vi "Autonomous Independent.vi"() -> ()   [LabVIEW 2017]
doc: "This VI is called when autonomous begins, and will automatically be terminated when autonomous ends. You can carry out timed or sensor driven robot movement independently without needing to return to the caller."
uses:
  <vilib>/Rock Robotics/WPI/Utilities/WPI_GetSetVariantRefNum.vi
  <vilib>/Rock Robotics/Network Tables/NT Read String.vi
  <vilib>/Rock Robotics/Network Tables/NT Write Numeric Array.vi
  <vilib>/Rock Robotics/Network Tables/NT Write String.vi
  <vilib>/Rock Robotics/Network Tables/NT Write Number.vi
  <vilib>/Rock Robotics/Network Tables/NT Read Number.vi
  <vilib>/Rock Robotics/WPI/Ultrasonic/WPI_SonarMB1010AnalogRefNum Registry Get.vi
  <vilib>/addons/control/pid/NI_PID_pid.lvlib
  <vilib>/addons/control/pid/pid.llb/PID (DBL).vi
  <vilib>/Rock Robotics/WPI/Ultrasonic/WPI_SonarMB1010AnalogGetRange.vi
panel:
  out "Current Movement, for debugging":T1 {"Y Joystick Value" scale=1.0..-1.0; "X Joystick Value" scale=-1.0..1.0}
  in  "Array of robot movements":T2(array[cluster])=[{"X Joystick Value"=0.39393939393939403, "Y Joystick Value"=0.0, "Delay (sec)"=1.0, "Movement Name"="turn"}, {"X Joystick Value"=-0.3737373737373737, "Y Joystick Value"=0.0, "Delay (sec)"=1.0, "Movement Name"="turn back"}] {"Y Joystick Value" scale=1.0..-1.0; "X Joystick Value" scale=-1.0..1.0}
  # "Be sure to right-click and choose Data Operations>>Make Current Value default if you want to save the array values with the VI"
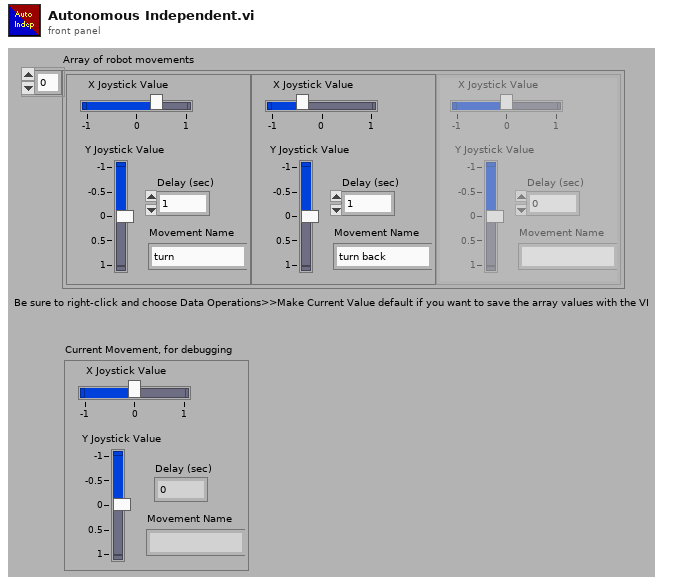
[diagram p1: front panel]
types:
  T1 = cluster{"X Joystick Value":dbl, "Y Joystick Value":dbl, "Delay (sec)":dbl, "Movement Name":string}
  T2 = cluster{"X Joystick Value":dbl, "Y Joystick Value":dbl, "Delay (sec)":dbl, "Movement Name":string}[]
  T3 = typedef "NetComm_MatchType.ctl" = enum32{"None", "Practice", "Qualification", "Elimination"}
  T4 = typedef "WPI_DriverStationPositionInfo.ctl" = enum16{"1", "2", "3"}
  T5 = typedef "WPI_DriverStationAllianceInfo.ctl" = enum16{"Red", "Blue", "Invalid"}
  T6 = typedef "WPI_JoystickDevRef.ctl" = cluster{"Device":T7}
  T7 = typedef "WPI_JoystickDeviceEnum.ctl" = enum16{"USB 0", "USB 1", "USB 2", "USB 3", "USB 4", "USB 5"}
  T8 = typedef "WPI_GyroDevRef.ctl" = cluster{"DevStatus":errorcluster, "Analog Channel":T9, "Gain (VoltsPerDegree/Second)":dbl, "Gyro Type":enum16{"Analog", "XRS450"}, "Handle":i32, "SPI Bus":T10, "Device Found":bool, "Sample Rate":dbl, "Calibrate On Open":bool, "Offset":dbl}
  T9 = typedef "FPGA_AIChannel.ctl" = enum8{"AI 0", "AI 1", "AI 2", "AI 3", "AI MXP 0", "AI MXP 1", "AI MXP 2", "AI MXP 3", "Invalid"}
  T10 = typedef "spi_bus.ctl" = enum16{"SPI On-Board, CS0", "SPI On-Board, CS1", "SPI On-Board, CS2", "SPI On-Board, CS3", "SPI MXP", "Invalid"}
  T11 = typedef "WPI_RobotDriveDevRef.ctl" = cluster{"DevStatus":errorcluster, "Motors[]":T12[], "Square Inputs":bool, "Max Output":dbl}
  T12 = typedef "WPI_MotorControlDeviceRef.ctl" = cluster{"DeviceStatus":errorcluster, "Type":T13, "PWM":cluster{"PWM Channel":T14, "DeadBand":T15}, "CAN":cluster{"Device Number":u8, "SetOutput VI Ref":variant, "GetOutput VI Ref":variant, "Enable VI Ref":variant, "Disable VI Ref":variant, "Data":variant}, "Invert":bool, "DIO PWM":cluster{"PWM \"Enable\" Channel":T14, "DIOChannel":T16, "PWM Rate":dbl}}
  T13 = typedef "WPI_MotorControlType.ctl" = enum16{"PWM", "CAN", "DIO PWM"}
  T14 = typedef "FPGA_DIOPWMChannel.ctl" = enum8{"PWM 0", "PWM 1", "PWM 2", "PWM 3", "PWM 4", "PWM 5", "PWM 6", "PWM 7", "PWM 8", "PWM 9", "PWM MXP 0", "PWM MXP 1", "PWM MXP 2", "PWM MXP 3", "PWM MXP 4", "PWM MXP 5", "PWM MXP 6", "PWM MXP 7", "PWM MXP 8", "PWM MXP 9", "Invalid"}
  T15 = typedef "WPI_PWMDeadband.ctl" = cluster{"Name":string, "maxPositivePwm":i32, "minPositivePwm":i32, "centerPwm":i32, "maxNegativePwm":i32, "minNegativePwm":i32, "angularRange":u16}
  T16 = typedef "FPGA_DIOChannel.ctl" = enum8{"DIO 0", "DIO 1", "DIO 2", "DIO 3", "DIO 4", "DIO 5", "DIO 6", "DIO 7", "DIO 8", "DIO 9", "DIO MXP 0", "DIO MXP 1", "DIO MXP 2", "DIO MXP 3", "DIO MXP 4", "DIO MXP 5", "DIO MXP 6", "DIO MXP 7", "DIO MXP 8", "DIO MXP 9", "DIO MXP 10", "DIO MXP 11", "DIO MXP 12", "DIO MXP 13", "DIO MXP 14", "DIO MXP 15", "SPI Port CS1", "SPI Port CS2", "SPI Port CS3", "SPI Port MISO", "SPI Port MOSI", "Invalid"}
  T17 = typedef "WPI_SonarMB1010AnalogDeviceRef.ctl" = cluster{"AIDeviceRef":T18, "Scaling factor (V/in)":dbl, "Average Bits":u8}
  T18 = typedef "WPI_AnalogChannelDevRef.ctl" = cluster{"DevStatus":errorcluster, "Analog Channel":T9}
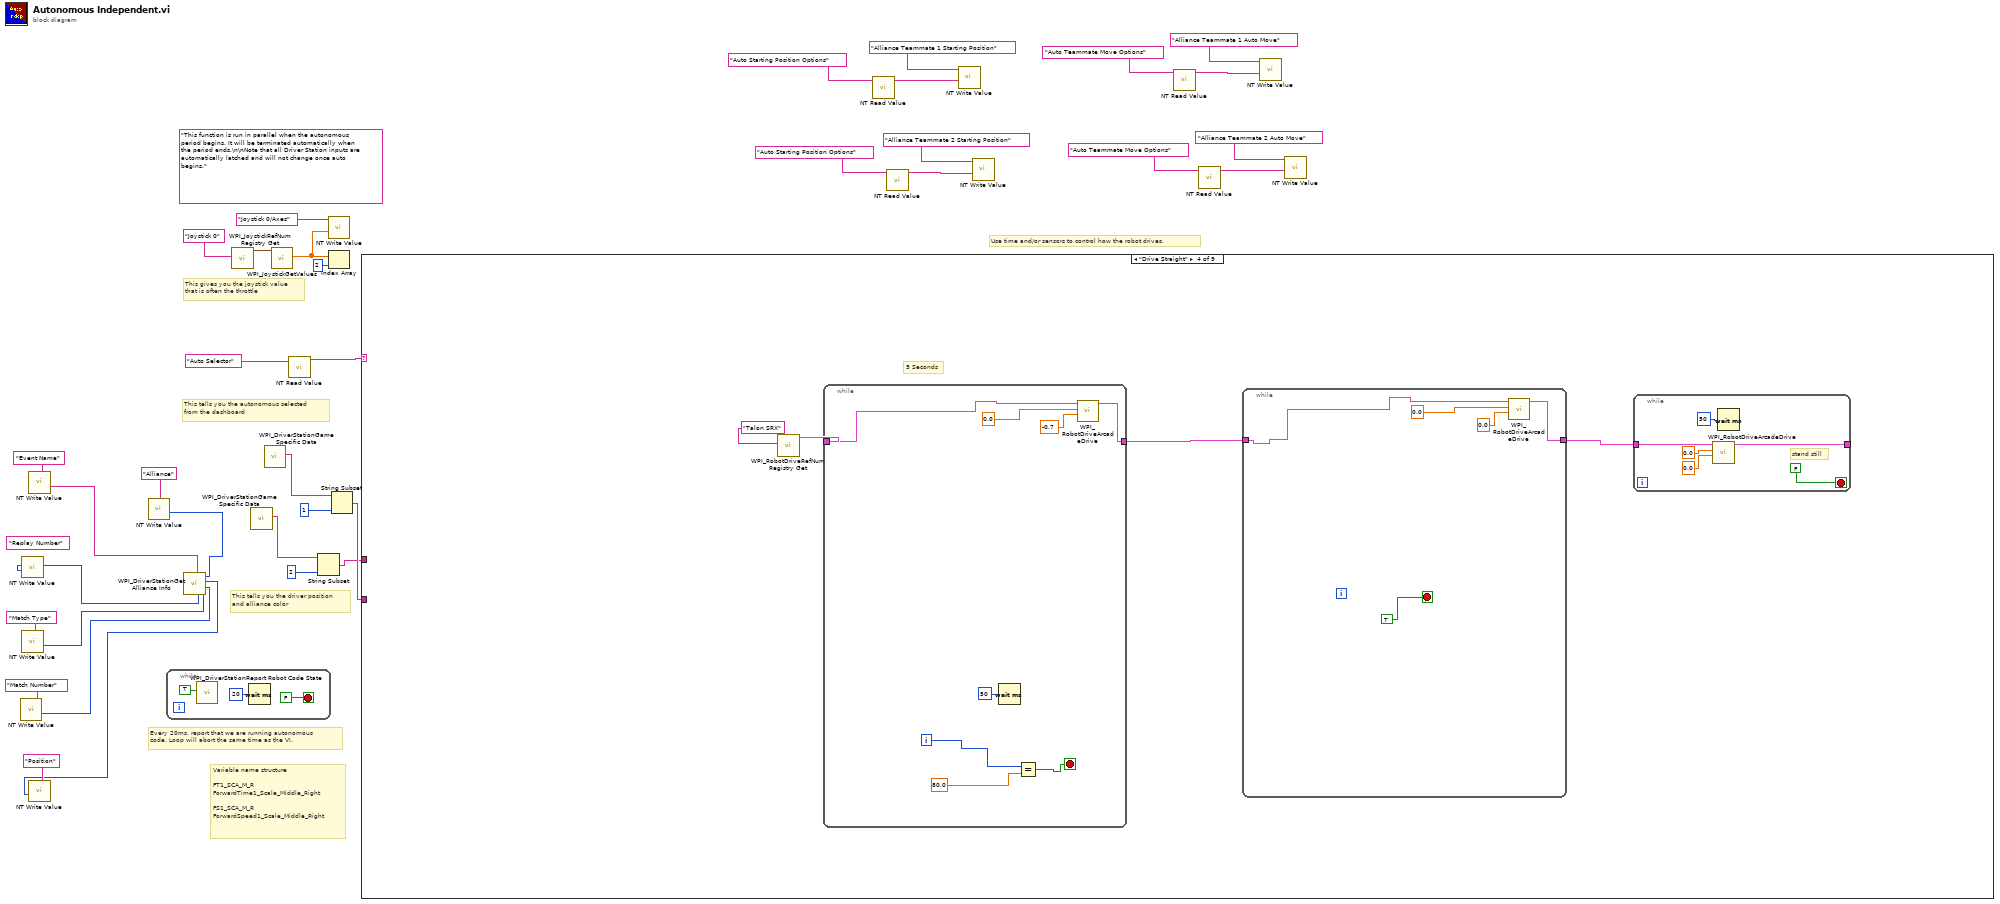
[diagram p0: block diagram]
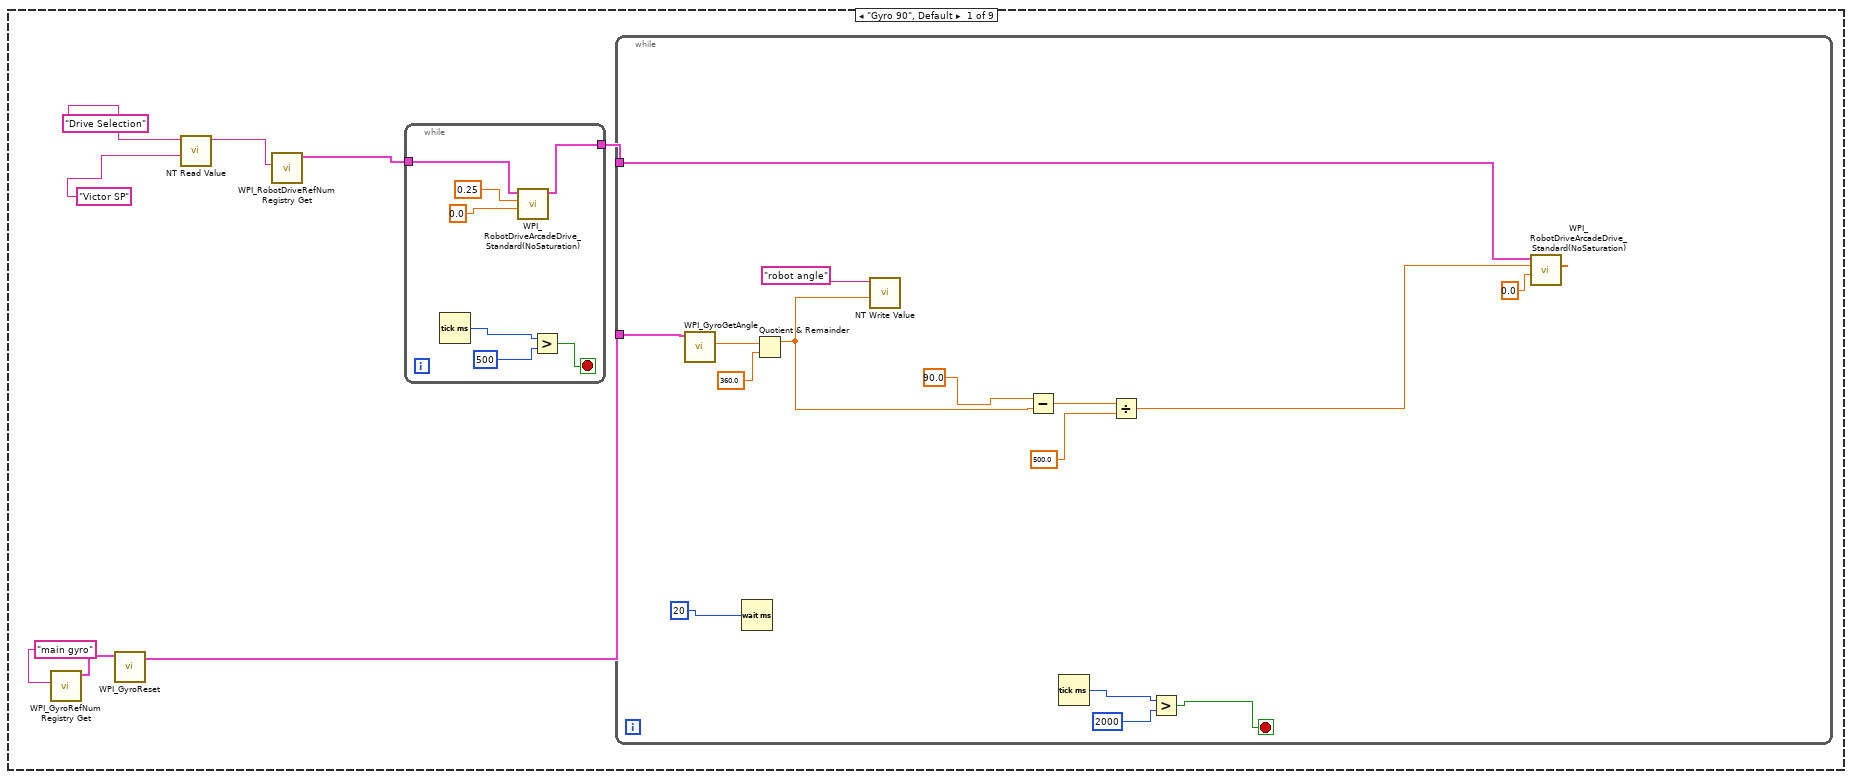
[diagram p2: hidden frame]
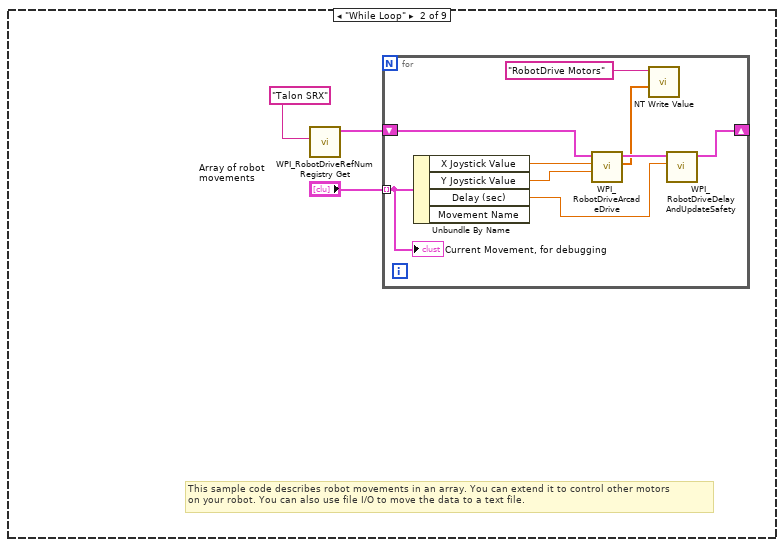
[diagram p3: hidden frame]
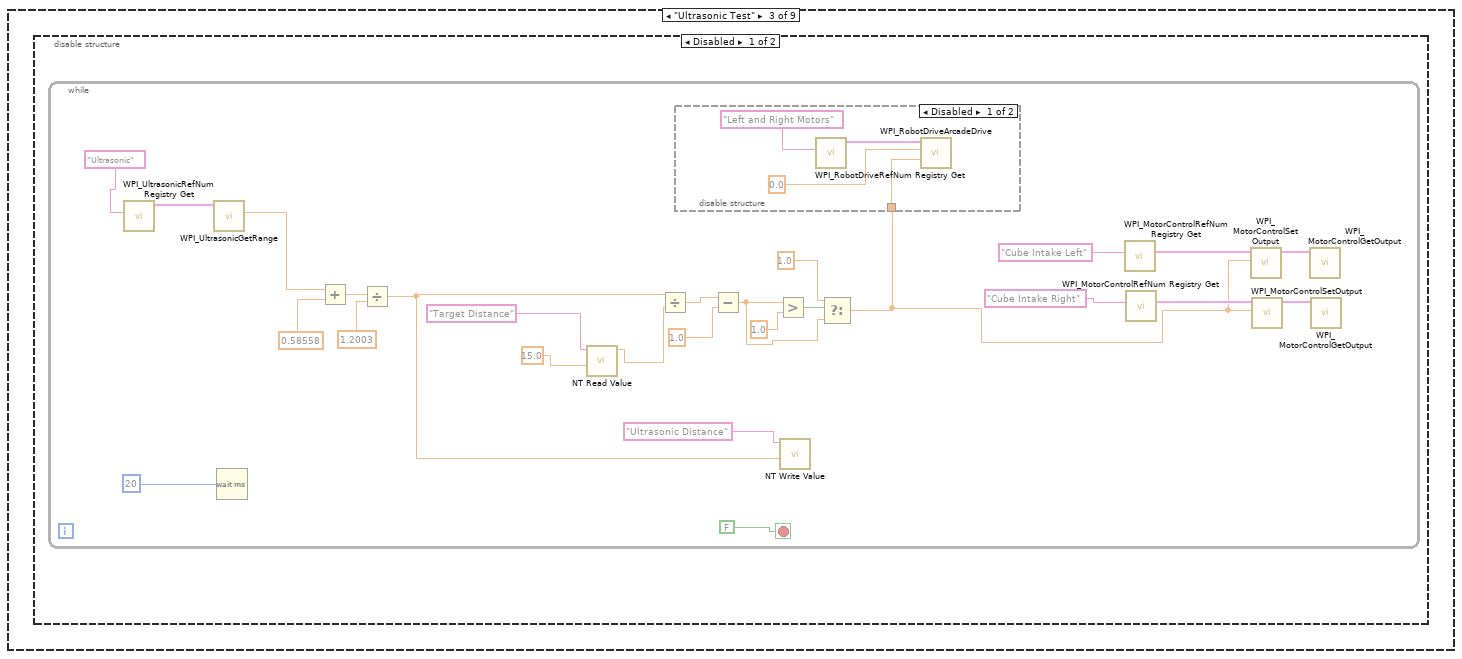
[diagram p4: hidden frame]
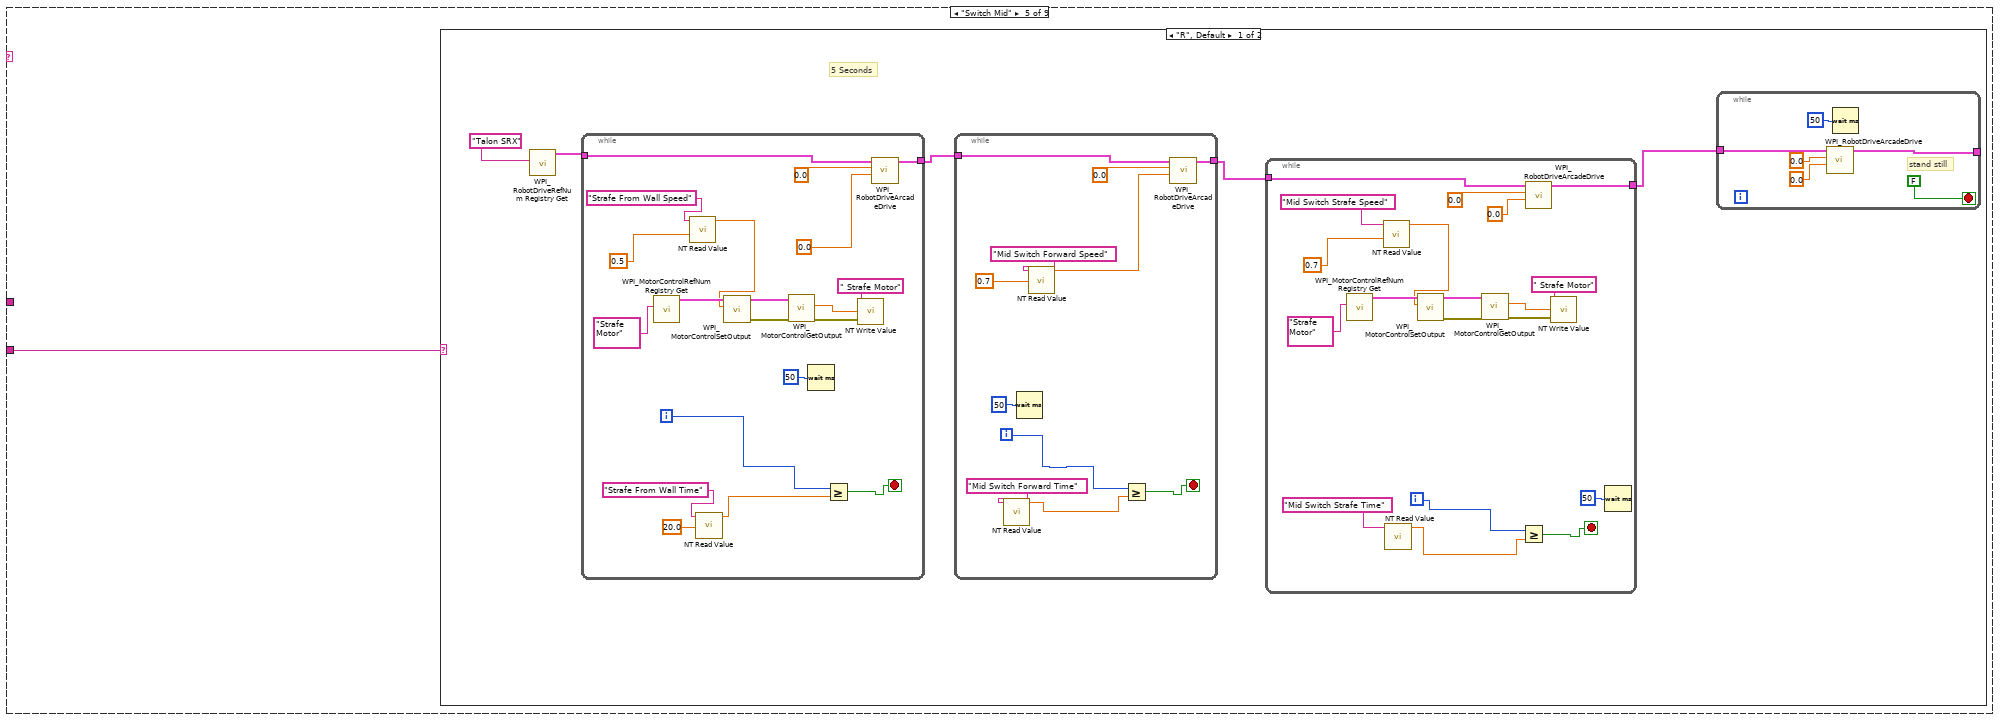
[diagram p7: hidden frame]
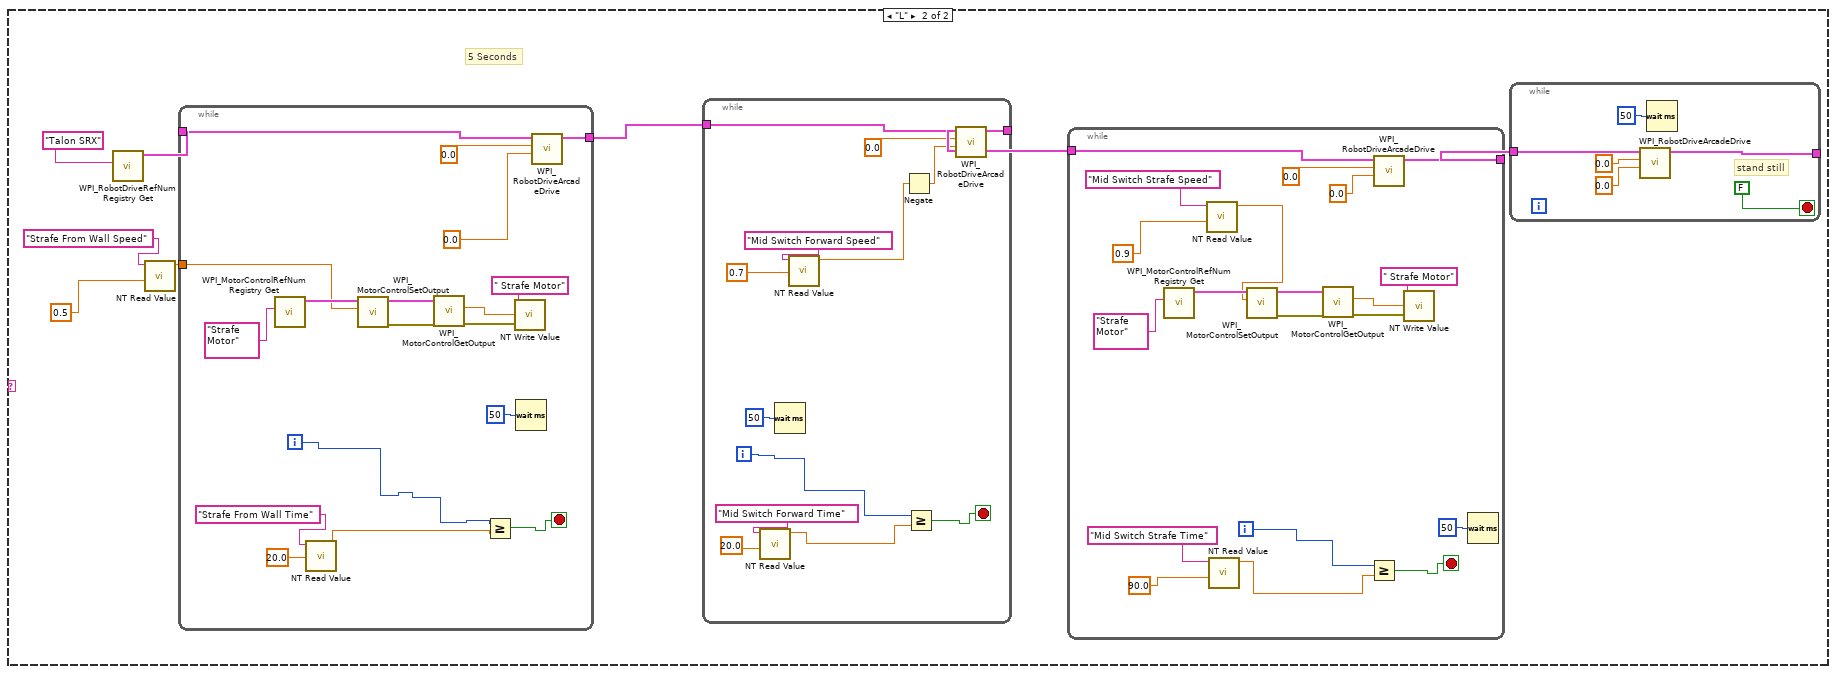
[diagram p8: hidden frame]
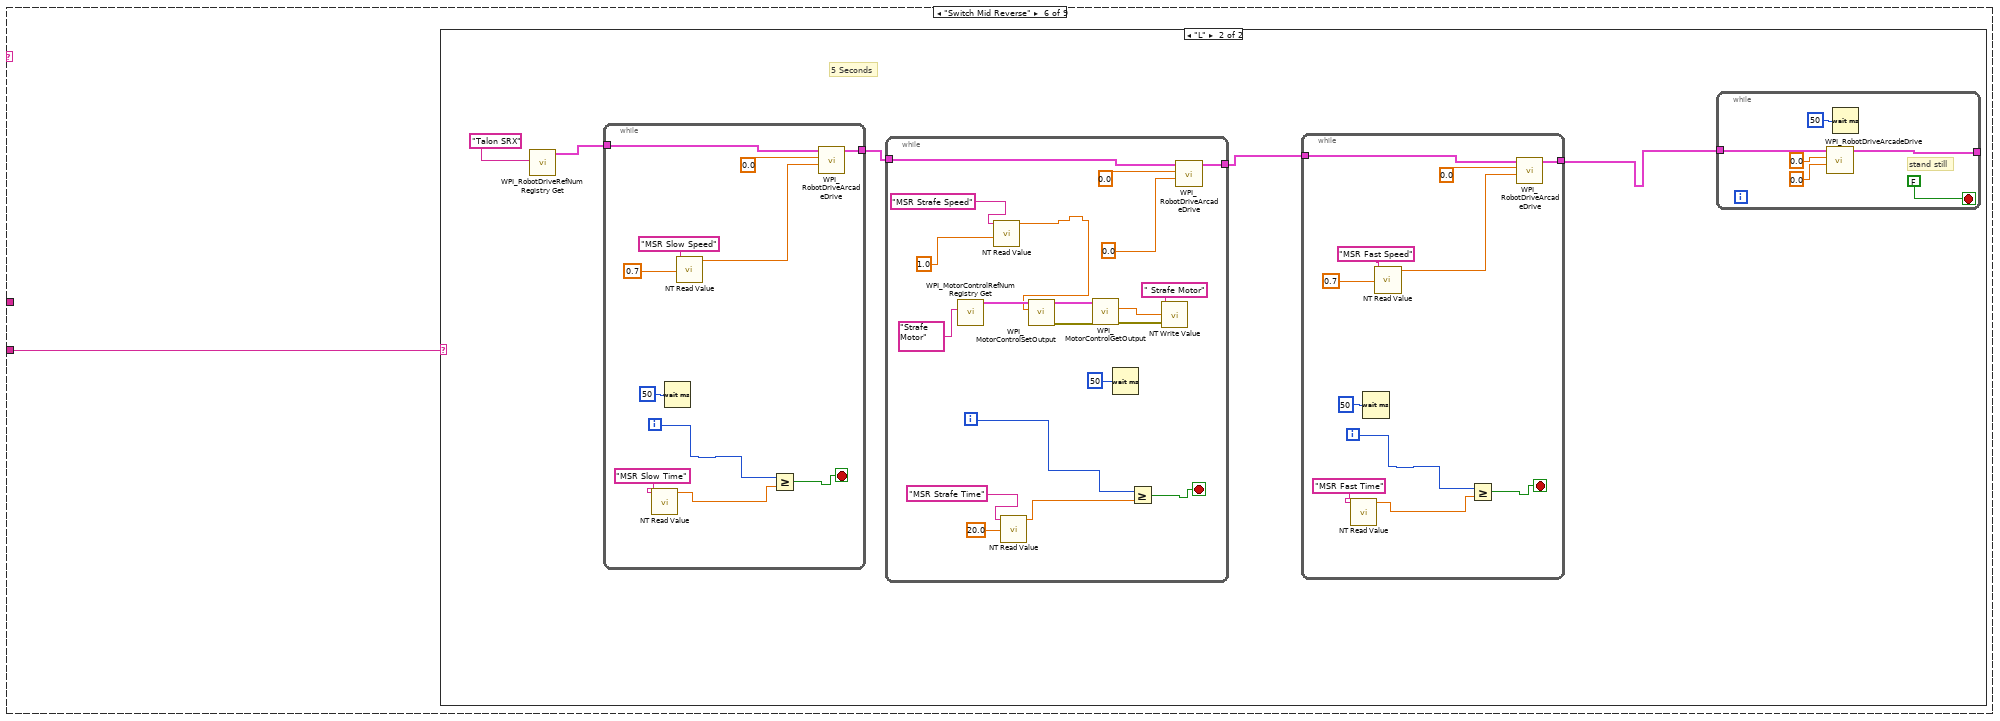
[diagram p9: hidden frame]
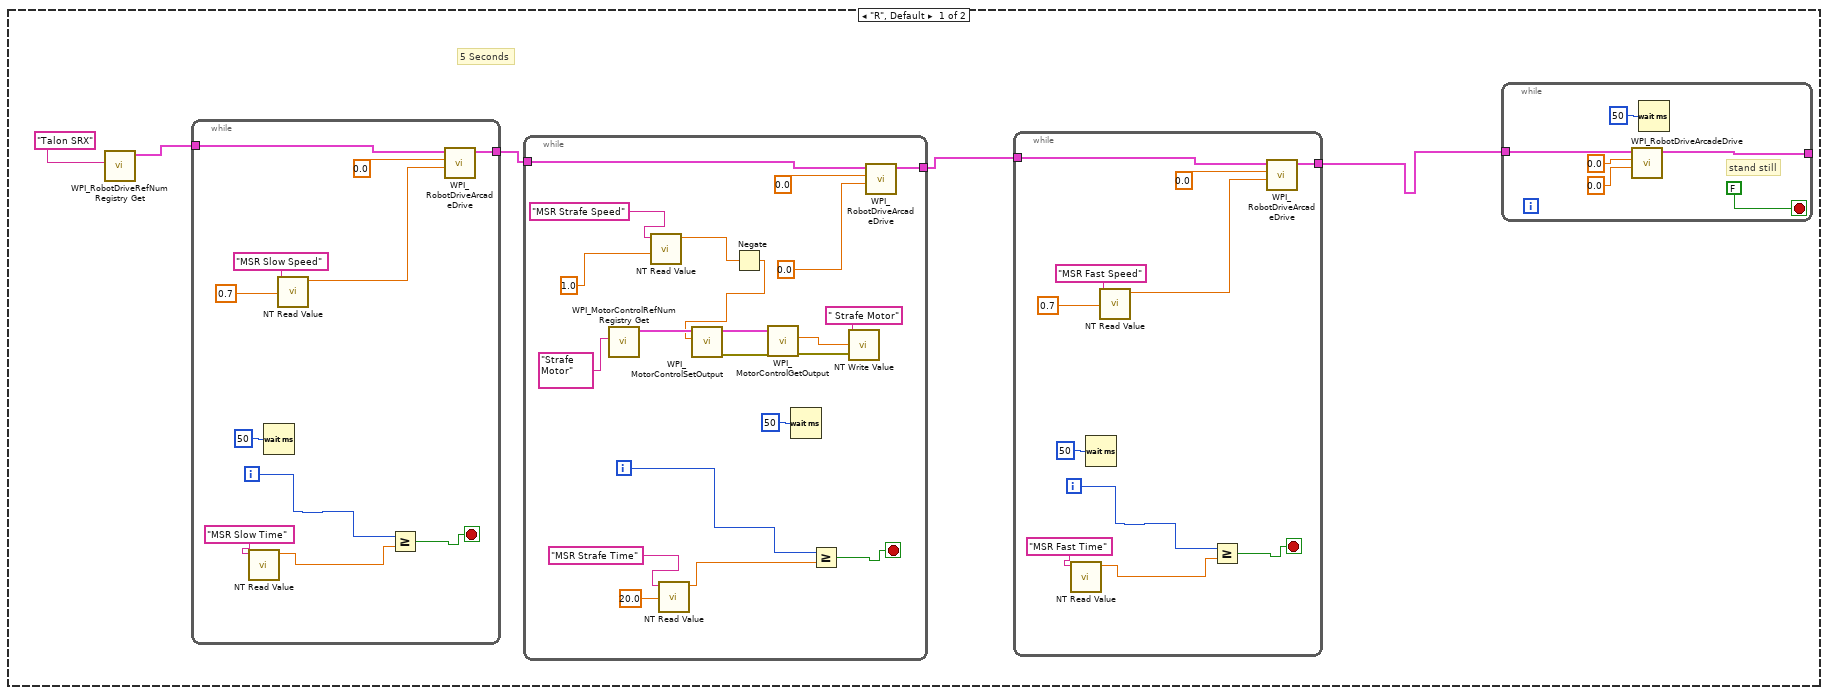
[diagram p10: hidden frame]
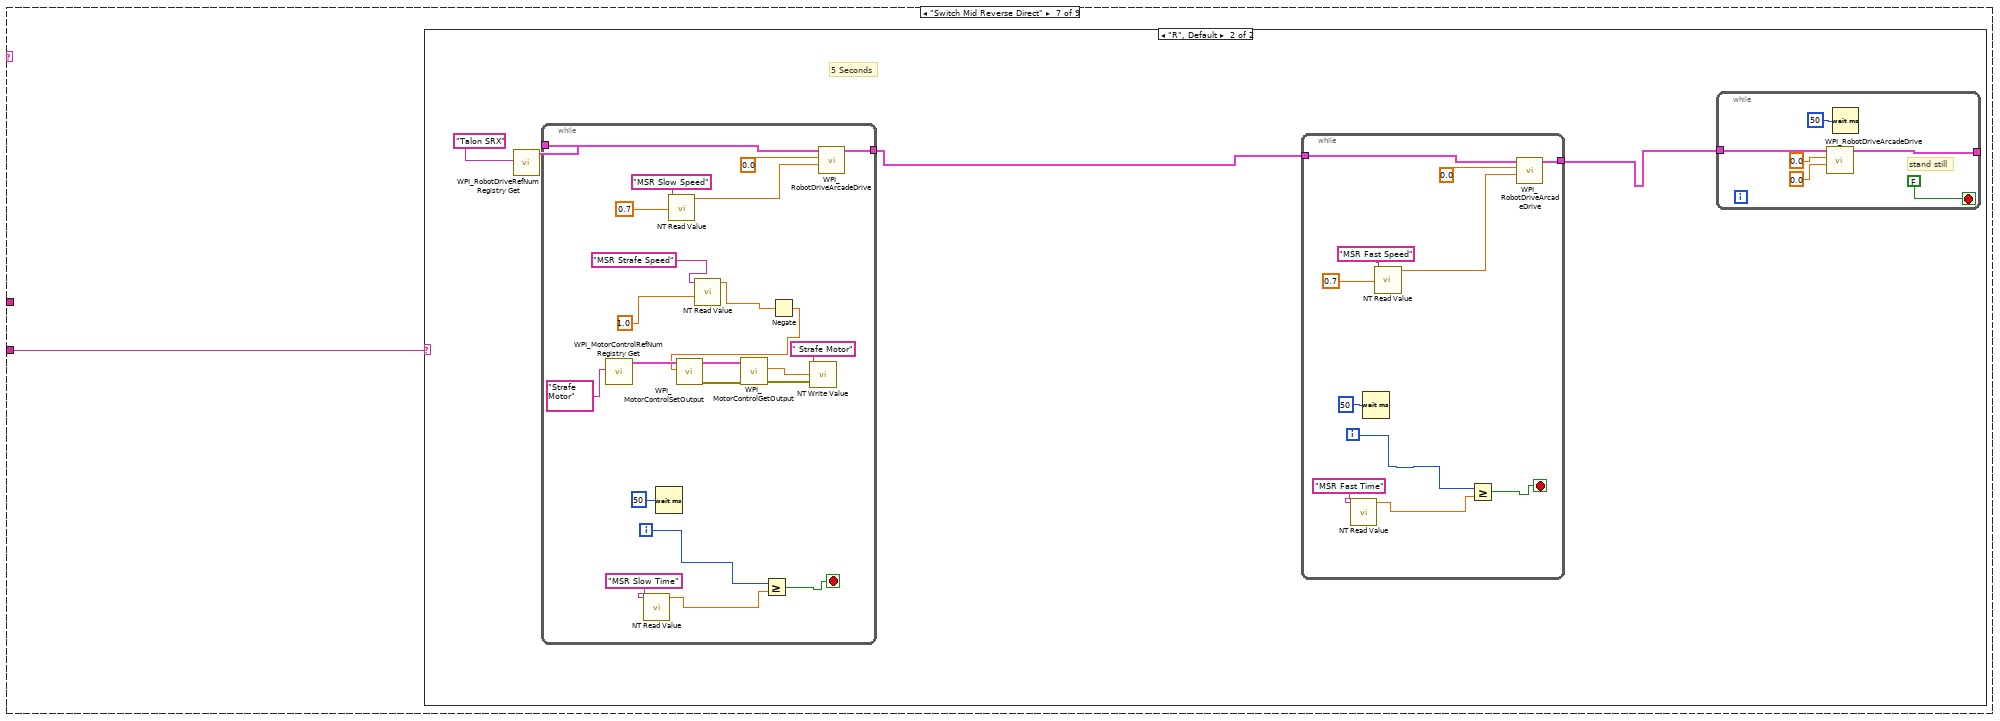
[diagram p11: hidden frame]
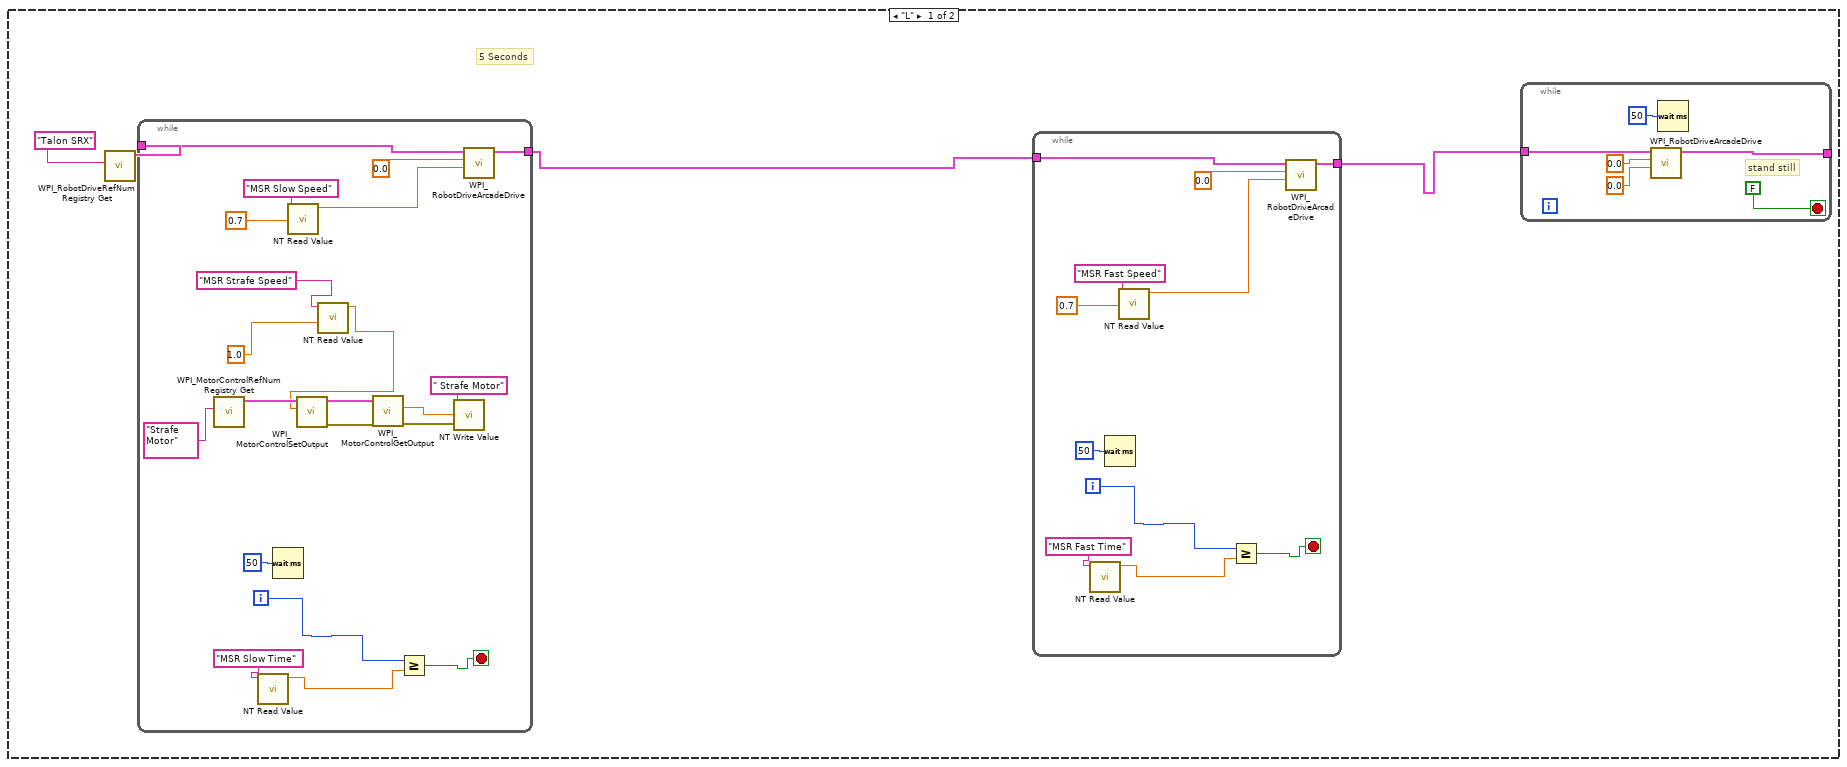
[diagram p12: hidden frame]
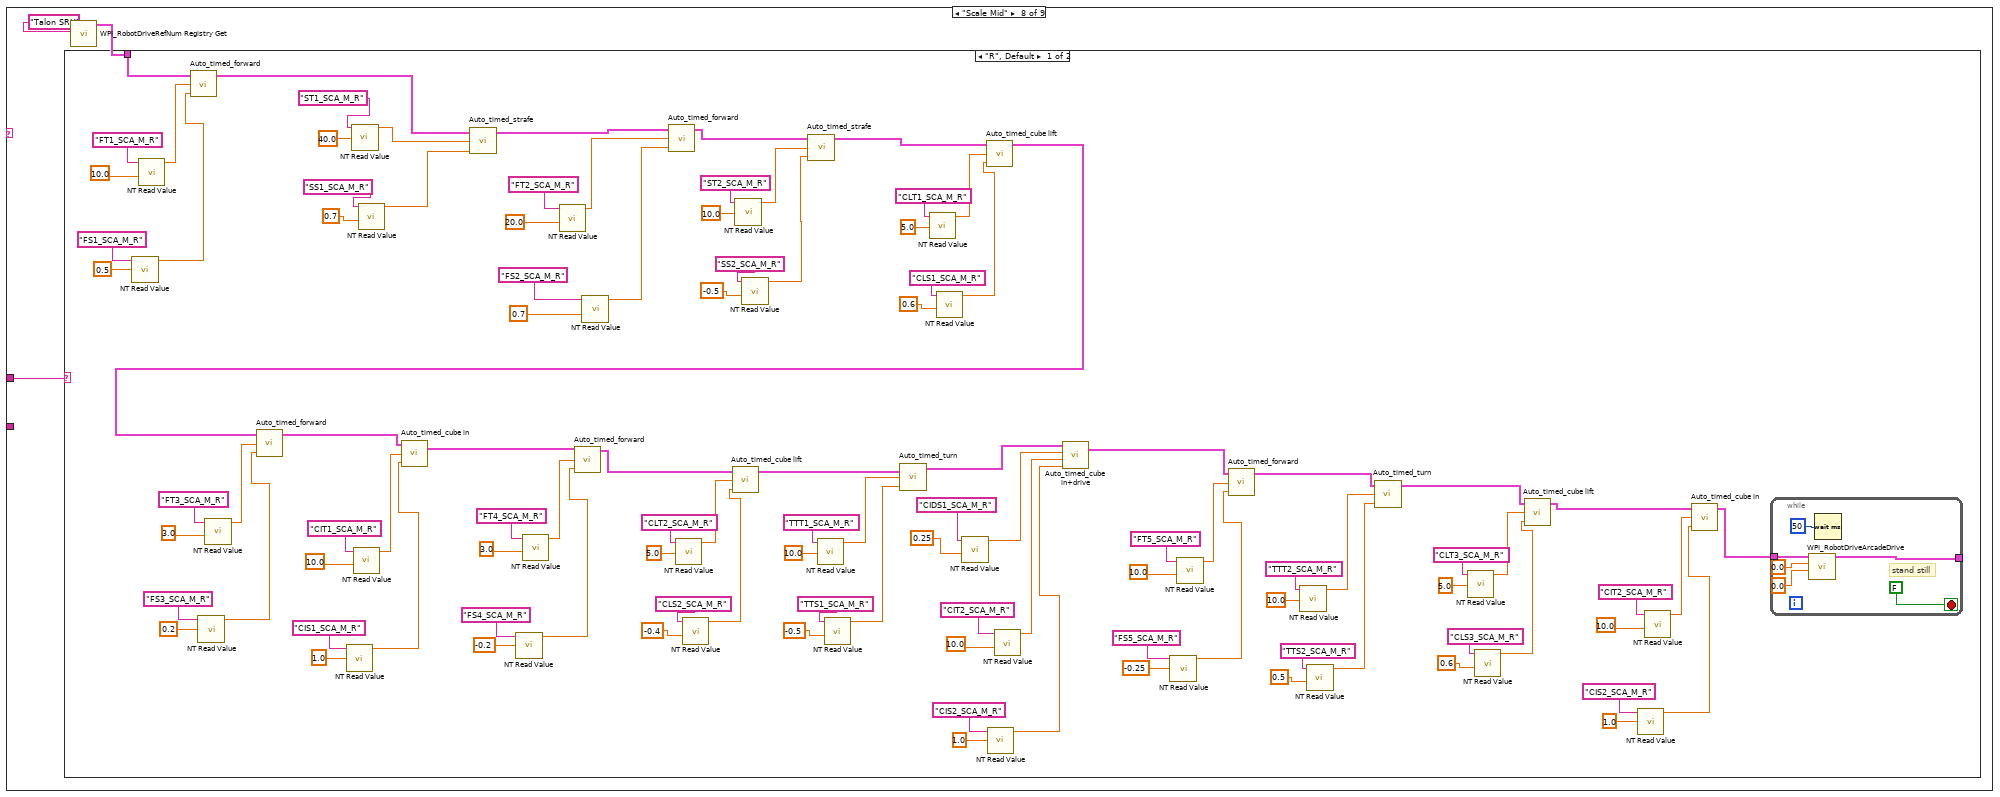
[diagram p13: hidden frame]
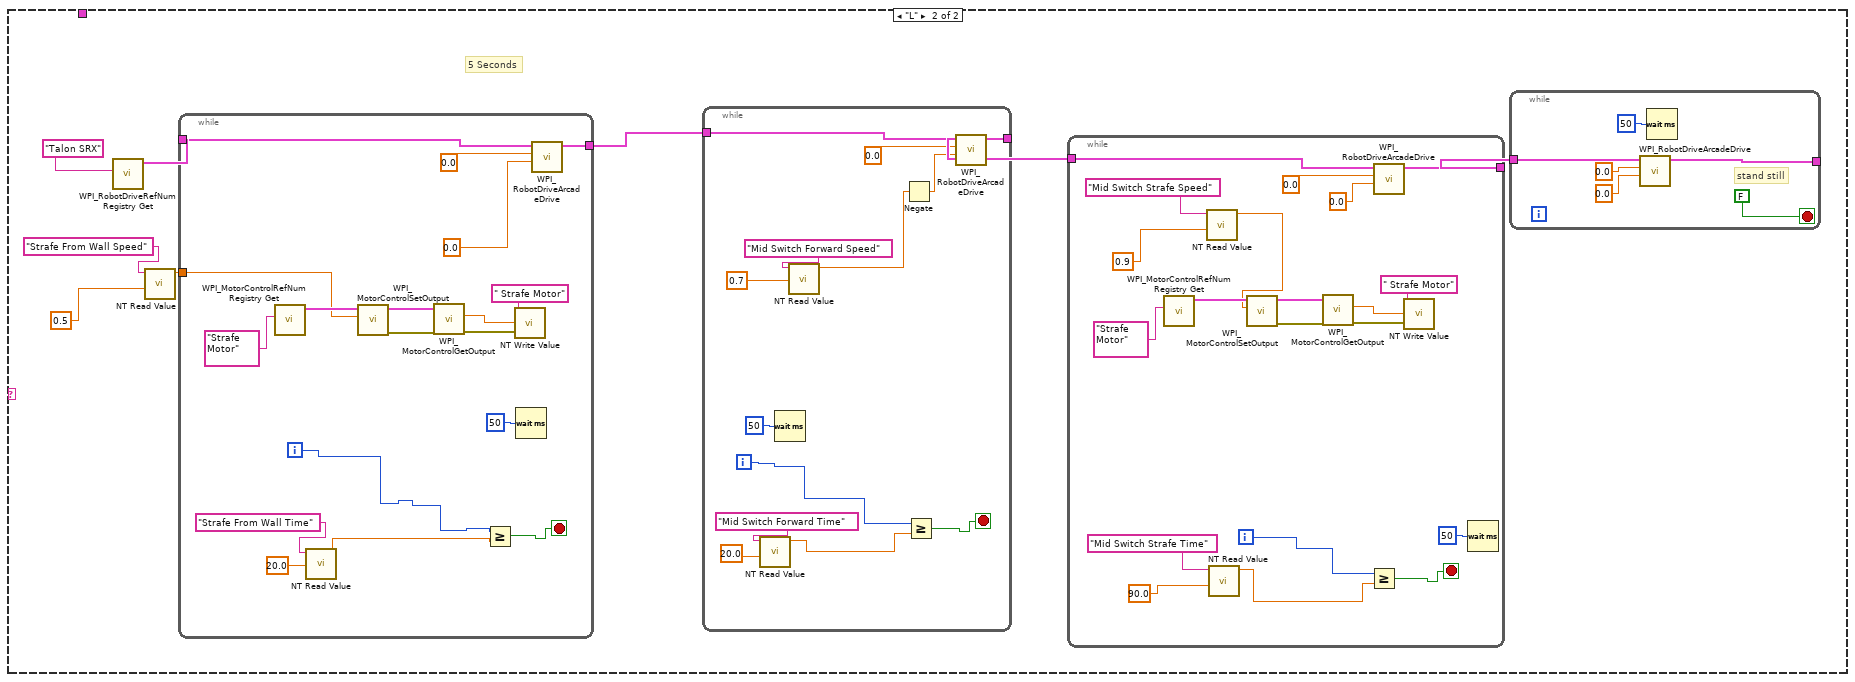
[diagram p14: hidden frame]
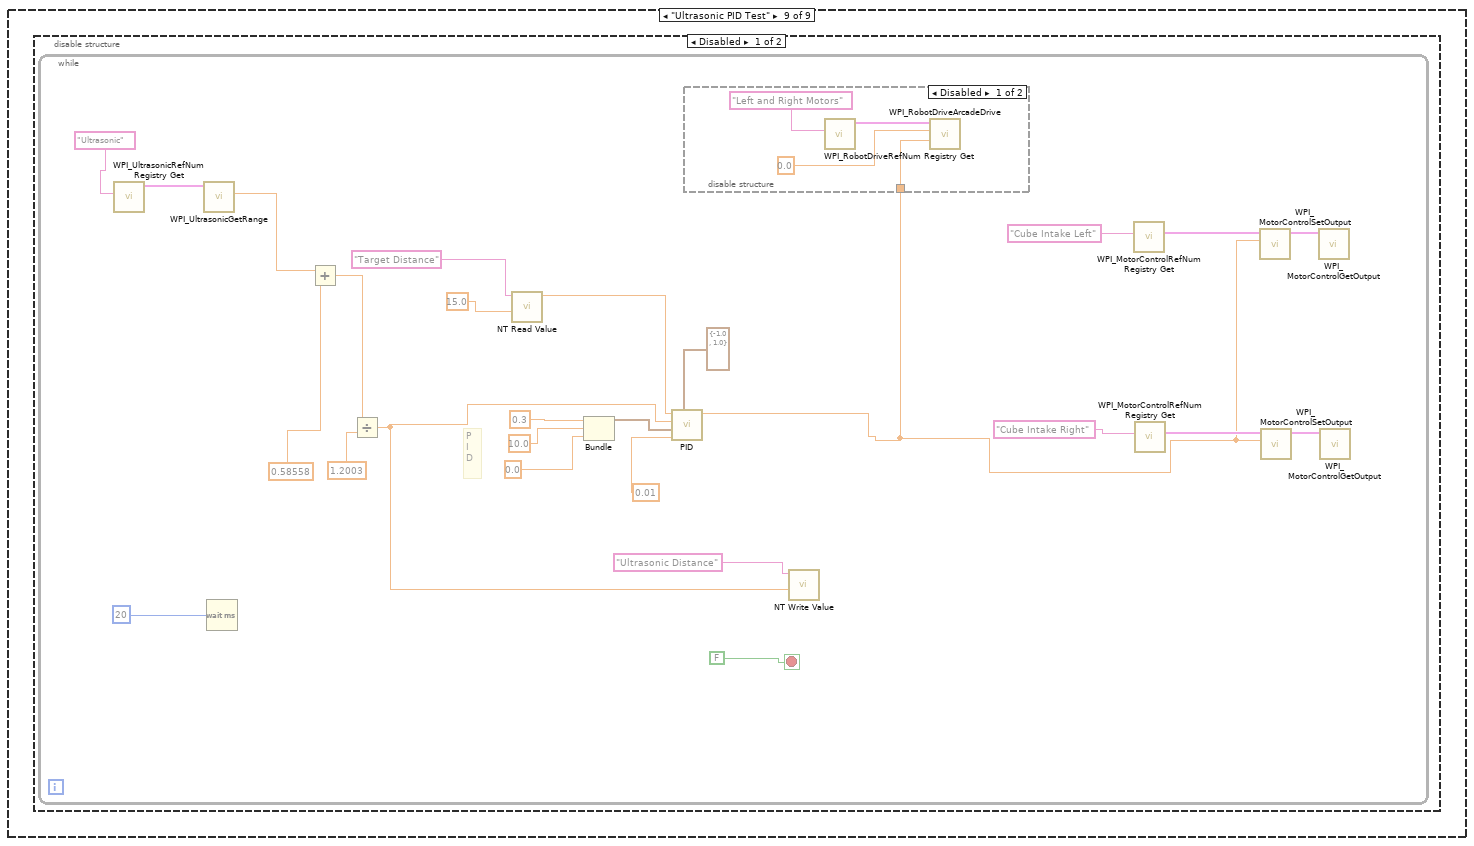
[diagram p15: hidden frame]
diagram:
  (unwired) "Replay Number"
  (unwired) "This function is run in parallel when the autonomous period begins. It will be terminated automatically when the period ends.\n\nNote that all Driver Station inputs are automatically latched and will not change once auto begins."
  # "Variable name structure\n\nFT1_SCA_M_R\nForwardTime1_Scale_Middle_Right\n\nFS1_SCA_M_R\nForwardSpeed1_Scale_Middle_Right"
  # "This tells you the autonomous selected\nfrom the dashboard"
  # "Every 20ms, report that we are running autonomous\ncode. Loop will abort the same time as the VI."
  # "This gives you the joystick value\nthat is often the throttle"
  # "Use time and/or sensors to control how the robot drives."
  # "This tells you the driver position\nand alliance color"
  n1 = while {
    stop <- FALSE stop-if-true
    n2 = call <vilib>:"WPI_DriverStationReport Robot Code State.vi"("Autonomous"=TRUE) -> ()  [unwired: 10 in, 1 out]
    n3 = Wait (ms)(milliseconds to wait=u32 20) -> ()  [unwired: 1 out]
  }
  n4 = call <vilib>:"WPI_DriverStationGet Alliance Info.vi"() -> ("Match Type"=w17:T3, "Match Number"=w18:u16, "Position"=w19:T4, "Alliance"=w23:T5, "Replay Number"=w16:u16, "Event Name"=w25:string)  [unwired: 6 out]
  n5 = call-poly <vilib>:"NT Write Value.vi"("Numeric"=w18, "Name"="Match Number") -> ()  [unwired: 9 in, 1 out]
  n6 = call-poly <vilib>:"NT Write Value.vi"("Numeric"=w16) -> ()  [unwired: 10 in, 1 out]
  n7 = call-poly <vilib>:"NT Write Value.vi"("Numeric"=w17, "Name"="Match Type") -> ()  [unwired: 9 in, 1 out]
  n8 = call-poly <vilib>:"NT Write Value.vi"("String"=w25, "Name"="Event Name") -> ()  [unwired: 9 in, 1 out]
  n9 = call-poly <vilib>:"NT Write Value.vi"("Numeric"=w19, "Name"="Position") -> ()  [unwired: 9 in, 1 out]
  n10 = call-poly <vilib>:"NT Write Value.vi"("Numeric"=w23, "Name"="Alliance") -> ()  [unwired: 9 in, 1 out]
  n11 = call <vilib>:"WPI_JoystickRefNum Registry Get.vi"("refnum name"="Joystick 0") -> ("JoystickDevRef"=w35:T6)  [unwired: 1 in, 9 out]
  n12 = call <vilib>:"WPI_DriverStationGame Specific Data.vi"() -> ("Game Specific Data"=w3:string)  [unwired: 11 in]
  n13 = call <vilib>:"WPI_DriverStationGame Specific Data.vi"() -> ("Game Specific Data"=w29:string)  [unwired: 11 in]
  n14 = call <vilib>:"WPI_JoystickGetValues.vi"("JoystickDevRef"=w35) -> ("Axes"=w31:dbl[])  [unwired: 6 in, 4 out]
  n15 = call-poly <vilib>:"NT Read Value.vi"("Name"="Auto Selector") -> ("String"=w32:string)  [unwired: 9 in, 1 out]
  n16 = String Subset(string=w3, length (rest)=2 ("index")) -> (substring=w1:string)  [unwired: 1 in]
  n17 = call-poly <vilib>:"NT Write Value.vi"("Numeric Array"=w31, "Name"="Joystick 0/Axes") -> ()  [unwired: 9 in, 1 out]
  n18 = Index Array(array=w31, index=2) -> ()  [unwired: 1 out]
  n19 = String Subset(string=w29, length (rest)=1 ("index")) -> (substring=w28:string)  [unwired: 1 in]
  n20 = case shown="\"Drive Straight\"" w32 {
    tunnel: w28 -> [_ _ _ _ w135 w262 w370 _ _]
    tunnel: w1 -> [_ _ _ _ _ _ _ w456 _]
    frame "Gyro 90", Default {
      n21 = call <vilib>:"WPI_GyroRefNum Registry Get.vi"("refnum name"="main gyro") -> ("GyroDevRef"=w45:T8)  [unwired: 9 in, 1 out]
      n22 = call <vilib>:"WPI_GyroReset.vi"("GyroDevRef"=w45) -> ("GyroDevRef"=w47:T8)  [unwired: 9 in, 1 out]
      n23 = call-poly <vilib>:"NT Read Value.vi"("Default Value"="Victor SP", "Name"="Drive Selection") -> ("String"=w44:string)  [unwired: 8 in, 1 out]
      n24 = call <vilib>:"WPI_RobotDriveRefNum Registry Get.vi"("refnum name"=w44) -> ("RobotDriveDevRef"=w41:T11)  [unwired: 1 in, 9 out]
      n25 = while {
        tunnel: w41 -> [w51]
        tunnel: [w48] -> w40
        stop <- w52 stop-if-true
        n26 = Tick Count (ms)() -> (millisecond timer value=w53:u32)
        n27 = call <vilib>:"WPI_RobotDriveArcadeDrive_Standard(NoSaturation).vi"("Y axis value"=0.0, "X axis value"=0.25, "RobotDriveDevRef"=w51) -> ("RobotDriveDevRef"=w48:T11)  [unwired: 1 in, 7 out]
        n28 = Greater?(x=w53, y=500) -> (0:w52:bool)
      }
      n29 = while {
        tunnel: w47 -> [w66]
        tunnel: w40 -> [w63]
        stop <- w62 stop-if-true
        n30 = call <vilib>:"WPI_GyroGetAngle.vi"("GyroDevRef"=w66) -> ("Angle"=w67:dbl)  [unwired: 6 in, 4 out]
        n31 = Wait (ms)(milliseconds to wait=u32 20) -> ()  [unwired: 1 out]
        n32 = Quotient & Remainder(x=w67, y=360.0) -> (x-y*floor(x/y)=w58:dbl)  [unwired: 1 out]
        n33 = call-poly <vilib>:"NT Write Value.vi"("Numeric"=w58, "Name"="robot angle") -> ()  [unwired: 9 in, 1 out]
        n34 = Subtract(x=90.0, y=w58) -> (x-y=w57:dbl)
        n35 = Tick Count (ms)() -> (millisecond timer value=w60:u32)
        n36 = Divide(x=w57, y=500.0) -> (x/y=w55:dbl)
        n37 = Greater?(x=w60, y=2000) -> (0:w62:bool)
        n38 = call <vilib>:"WPI_RobotDriveArcadeDrive_Standard(NoSaturation).vi"("Y axis value"=0.0, "X axis value"=w55, "RobotDriveDevRef"=w63) -> ()  [unwired: 1 in, 8 out]
      }
    }
    frame "While Loop" {
      # "This sample code describes robot movements in an array. You can extend it to control other motors\non your robot. You can also use file I/O to move the data to a text file."
      n39 = call <vilib>:"WPI_RobotDriveRefNum Registry Get.vi"("refnum name"="Talon SRX") -> ("RobotDriveDevRef"=w71:T11)  [unwired: 1 in, 9 out]
      n40 = for {
        shift-right: [w79] -> _
        shift-left: w71 -> [w80]
        tunnel: "Array of robot movements" -> [w75] mode=indexing
        n41 = Unbundle By Name(w75) -> ("X Joystick Value"=w78:dbl, "Y Joystick Value"=w77:dbl, "Delay (sec)"=w76:dbl)  [unwired: 1 out]
        n42 = call-poly <vilib>:"WPI_RobotDriveArcadeDrive.vi"("Y axis value"=w77, "X axis value"=w78, "RobotDriveDevRef"=w80) -> ("Motor Values"=w73:dbl[], "RobotDriveDevRef"=w81:T11)  [unwired: 1 in, 6 out]
        n43 = call-poly <vilib>:"NT Write Value.vi"("Numeric Array"=w73, "Name"="RobotDrive Motors") -> ()  [unwired: 9 in, 1 out]
        n44 = call <vilib>:"WPI_RobotDriveDelayAndUpdateSafety.vi"("Delay (s)"=w76, "RobotDriveDevRef"=w81) -> ("RobotDriveDevRef 2"=w79:T11)  [unwired: 8 in, 1 out]
        "Current Movement, for debugging" <- w75
      }
    }
    frame "Ultrasonic Test" {
      n45 = disable-structure shown="Disabled" {
        frame Disabled {
          n46 = while {
            stop <- FALSE stop-if-true
            n47 = call-poly <vilib>:"WPI_UltrasonicRefNum Registry Get.vi"("refnum name"="Ultrasonic") -> ("SonarMB1010AnalogDevRef"=w106:T17)  [unwired: 9 in, 1 out]
            n48 = call-poly <vilib>:"WPI_UltrasonicGetRange.vi"("SonarMB1010AnalogDevRef"=w106) -> ("Distance"=w105:dbl)  [unwired: 8 in, 2 out]
            n49 = Wait (ms)(milliseconds to wait=u32 20) -> ()  [unwired: 1 out]
            n50 = Add(x=w105, y=0.58558) -> (x+y=w103:dbl)
            n51 = Divide(x=w103, y=1.2003) -> (x/y=w95:dbl)
            n52 = call-poly <vilib>:"NT Read Value.vi"("Default Value"=15.0, "Name"="Target Distance" ("refnum name")) -> ("Numeric"=w85:dbl)  [unwired: 8 in, 1 out]
            n53 = Divide(x=w95, y=w85) -> (x/y=w100:dbl)
            n54 = Subtract(x=w100, y=1.0) -> (x-y=w96:dbl)
            n55 = Greater?(x=w96, y=1.0) -> (0:w99:bool)
            n56 = call-poly <vilib>:"NT Write Value.vi"("Numeric"=w95, "Name"="Ultrasonic Distance" ("refnum name")) -> ()  [unwired: 9 in, 1 out]
            n57 = Select(t=1.0, s=w99, f=w96) -> (s? t:f=w86:dbl)
            n58 = disable-structure shown="Disabled" {
              disable-tunnel: w86 -> [w108 _]
              frame Disabled {
                n59 = call <vilib>:"WPI_RobotDriveRefNum Registry Get.vi"("refnum name"="Left and Right Motors") -> ("RobotDriveDevRef"=w110:T11)  [unwired: 1 in, 9 out]
                n60 = call-poly <vilib>:"WPI_RobotDriveArcadeDrive.vi"("Y axis value"=w108, "X axis value"=0.0, "RobotDriveDevRef"=w110) -> ()  [unwired: 1 in, 8 out]
              }
              frame Enabled {
              }
            }
            n61 = call <vilib>:"WPI_MotorControlRefNum Registry Get.vi"("refnum name"="Cube Intake Left") -> ("MotorControlDevRef"=w89:T12)  [unwired: 9 in, 1 out]
            n62 = call <vilib>:"WPI_MotorControlRefNum Registry Get.vi"("refnum name"="Cube Intake Right") -> ("MotorControlDevRef"=w92:T12)  [unwired: 9 in, 1 out]
            n63 = call <vilib>:"WPI_MotorControlSetOutput.vi"("Output"=w86, "MotorControlDevRef"=w89) -> ("MotorControlDevRef"=w90:T12)  [unwired: 7 in, 2 out]
            n64 = call <vilib>:"WPI_MotorControlSetOutput.vi"("Output"=w86, "MotorControlDevRef"=w92) -> ("MotorControlDevRef"=w91:T12)  [unwired: 7 in, 2 out]
            n65 = call <vilib>:"WPI_MotorControlGetOutput.vi"("MotorControlDevRef"=w90) -> ()  [unwired: 8 in, 3 out]
            n66 = call <vilib>:"WPI_MotorControlGetOutput.vi"("MotorControlDevRef"=w91) -> ()  [unwired: 8 in, 3 out]
          }
        }
        frame Enabled {
        }
      }
    }
    frame "Drive Straight" {
      # "5 Seconds"
      n67 = call <vilib>:"WPI_RobotDriveRefNum Registry Get.vi"("refnum name"="Talon SRX") -> ("RobotDriveDevRef"=w114:T11)  [unwired: 1 in, 9 out]
      n68 = while {
        tunnel: w114 -> [w122]
        tunnel: [w121] -> w113
        i -> [w117]
        stop <- w116 stop-if-true
        n69 = Wait (ms)(milliseconds to wait=50) -> ()  [unwired: 1 out]
        n70 = Equal?(x=w117, y=80.0) -> (x = y?=w116:bool)
        n71 = call-poly <vilib>:"WPI_RobotDriveArcadeDrive.vi"("Y axis value"=-0.7 ("X axis value"), "X axis value"=0.0, "RobotDriveDevRef"=w122) -> ("RobotDriveDevRef"=w121:T11)  [unwired: 1 in, 7 out]
      }
      n72 = while {
        tunnel: w113 -> [w133]
        tunnel: [w132] -> w112
        stop <- TRUE stop-if-true
        n73 = call-poly <vilib>:"WPI_RobotDriveArcadeDrive.vi"("Y axis value"=0.0 ("X axis value"), "X axis value"=0.0, "RobotDriveDevRef"=w133) -> ("RobotDriveDevRef"=w132:T11)  [unwired: 1 in, 7 out]
      }
      n74 = while {
        tunnel: w112 -> [w125]
        tunnel: [w124] -> _
        stop <- FALSE stop-if-true
        # "stand still"
        n75 = call-poly <vilib>:"WPI_RobotDriveArcadeDrive.vi"("Y axis value"=0.0 ("X axis value"), "X axis value"=0.0, "RobotDriveDevRef"=w125) -> ("RobotDriveDevRef"=w124:T11)  [unwired: 1 in, 7 out]
        n76 = Wait (ms)(milliseconds to wait=50) -> ()  [unwired: 1 out]
      }
    }
    frame "Switch Mid" {
      n77 = case shown="\"R\", Default" w135 {
        frame "R", Default {
          # "5 Seconds"
          n78 = call <vilib>:"WPI_RobotDriveRefNum Registry Get.vi"("refnum name"="Talon SRX") -> ("RobotDriveDevRef"=w137:T11)  [unwired: 1 in, 9 out]
          n79 = while {
            tunnel: [w160] -> w136
            tunnel: w137 -> [w156]
            i -> [w147]
            stop <- w159 stop-if-true
            n80 = call <vilib>:"WPI_MotorControlRefNum Registry Get.vi"("refnum name"="Strafe Motor") -> ("MotorControlDevRef"=w153:T12)  [unwired: 9 in, 1 out]
            n81 = call-poly <vilib>:"NT Read Value.vi"("Default Value"=0.5 ("X axis value"), "Name"="Strafe From Wall Speed") -> ("Numeric"=w141:dbl)  [unwired: 8 in, 1 out]
            n82 = call-poly <vilib>:"NT Read Value.vi"("Default Value"=20.0 ("X axis value"), "Name"="Strafe From Wall Time") -> ("Numeric"=w144:dbl)  [unwired: 8 in, 1 out]
            n83 = call <vilib>:"WPI_MotorControlSetOutput.vi"("Output"=w141, "MotorControlDevRef"=w153) -> ("error out"=w151:errorcluster, "MotorControlDevRef"=w152:T12)  [unwired: 7 in, 1 out]
            n84 = call <vilib>:"WPI_MotorControlGetOutput.vi"("error in"=w151, "MotorControlDevRef"=w152) -> ("error out"=w149:errorcluster, "Output"=w148:dbl)  [unwired: 7 in, 1 out]
            n85 = Wait (ms)(milliseconds to wait=50) -> ()  [unwired: 1 out]
            n86 = Greater Or Equal?(x=w147, y=w144) -> (x >= y?=w159:bool)
            n87 = call-poly <vilib>:"NT Write Value.vi"("error in"=w149, "Numeric"=w148, "Name"=" Strafe Motor") -> ()  [unwired: 8 in, 1 out]
            n88 = call-poly <vilib>:"WPI_RobotDriveArcadeDrive.vi"("Y axis value"=0.0 ("X axis value"), "X axis value"=0.0, "RobotDriveDevRef"=w156) -> ("RobotDriveDevRef"=w160:T11)  [unwired: 1 in, 7 out]
          }
          n89 = while {
            tunnel: [w190] -> w139
            tunnel: w136 -> [w186]
            i -> [w180]
            stop <- w189 stop-if-true
            n90 = call-poly <vilib>:"NT Read Value.vi"("Name"="Mid Switch Forward Time") -> ("Numeric"=w185:dbl)  [unwired: 9 in, 1 out]
            n91 = Wait (ms)(milliseconds to wait=50) -> ()  [unwired: 1 out]
            n92 = call-poly <vilib>:"NT Read Value.vi"("Default Value"=0.7 ("X axis value"), "Name"="Mid Switch Forward Speed") -> ("Numeric"=w181:dbl)  [unwired: 8 in, 1 out]
            n93 = Greater Or Equal?(x=w180, y=w185) -> (x >= y?=w189:bool)
            n94 = call-poly <vilib>:"WPI_RobotDriveArcadeDrive.vi"("Y axis value"=w181, "X axis value"=0.0, "RobotDriveDevRef"=w186) -> ("RobotDriveDevRef"=w190:T11)  [unwired: 1 in, 7 out]
          }
          n95 = while {
            tunnel: [w178] -> w138
            tunnel: w139 -> [w174]
            i -> [w161]
            stop <- w177 stop-if-true
            n96 = call <vilib>:"WPI_MotorControlRefNum Registry Get.vi"("refnum name"="Strafe Motor") -> ("MotorControlDevRef"=w172:T12)  [unwired: 9 in, 1 out]
            n97 = call-poly <vilib>:"NT Read Value.vi"("Default Value"=0.7 ("X axis value"), "Name"="Mid Switch Strafe Speed") -> ("Numeric"=w162:dbl)  [unwired: 8 in, 1 out]
            n98 = call-poly <vilib>:"NT Read Value.vi"("Name"="Mid Switch Strafe Time") -> ("Numeric"=w165:dbl)  [unwired: 9 in, 1 out]
            n99 = call <vilib>:"WPI_MotorControlSetOutput.vi"("Output"=w162, "MotorControlDevRef"=w172) -> ("error out"=w170:errorcluster, "MotorControlDevRef"=w171:T12)  [unwired: 7 in, 1 out]
            n100 = call <vilib>:"WPI_MotorControlGetOutput.vi"("error in"=w170, "MotorControlDevRef"=w171) -> ("error out"=w168:errorcluster, "Output"=w167:dbl)  [unwired: 7 in, 1 out]
            n101 = Greater Or Equal?(x=w161, y=w165) -> (x >= y?=w177:bool)
            n102 = call-poly <vilib>:"WPI_RobotDriveArcadeDrive.vi"("Y axis value"=0.0 ("X axis value"), "X axis value"=0.0, "RobotDriveDevRef"=w174) -> ("RobotDriveDevRef"=w178:T11)  [unwired: 1 in, 7 out]
            n103 = call-poly <vilib>:"NT Write Value.vi"("error in"=w168, "Numeric"=w167, "Name"=" Strafe Motor") -> ()  [unwired: 8 in, 1 out]
            n104 = Wait (ms)(milliseconds to wait=50) -> ()  [unwired: 1 out]
          }
          n105 = while {
            tunnel: w138 -> [w192]
            tunnel: [w191] -> _
            stop <- FALSE stop-if-true
            # "stand still"
            n106 = call-poly <vilib>:"WPI_RobotDriveArcadeDrive.vi"("Y axis value"=0.0 ("X axis value"), "X axis value"=0.0, "RobotDriveDevRef"=w192) -> ("RobotDriveDevRef"=w191:T11)  [unwired: 1 in, 7 out]
            n107 = Wait (ms)(milliseconds to wait=50) -> ()  [unwired: 1 out]
          }
        }
        frame "L" {
          # "5 Seconds"
          n108 = call <vilib>:"WPI_RobotDriveRefNum Registry Get.vi"("refnum name"="Talon SRX") -> ("RobotDriveDevRef"=w201:T11)  [unwired: 1 in, 9 out]
          n109 = call-poly <vilib>:"NT Read Value.vi"("Default Value"=0.5 ("X axis value"), "Name"="Strafe From Wall Speed") -> ("Numeric"=w197:dbl)  [unwired: 8 in, 1 out]
          n110 = while {
            tunnel: [w222] -> w200
            tunnel: w201 -> [w219]
            tunnel: w197 -> [w210]
            i -> [w206]
            stop <- w207 stop-if-true
            n111 = call <vilib>:"WPI_MotorControlRefNum Registry Get.vi"("refnum name"="Strafe Motor") -> ("MotorControlDevRef"=w216:T12)  [unwired: 9 in, 1 out]
            n112 = call-poly <vilib>:"NT Read Value.vi"("Default Value"=20.0 ("X axis value"), "Name"="Strafe From Wall Time") -> ("Numeric"=w205:dbl)  [unwired: 8 in, 1 out]
            n113 = call <vilib>:"WPI_MotorControlSetOutput.vi"("Output"=w210, "MotorControlDevRef"=w216) -> ("error out"=w214:errorcluster, "MotorControlDevRef"=w215:T12)  [unwired: 7 in, 1 out]
            n114 = call <vilib>:"WPI_MotorControlGetOutput.vi"("error in"=w214, "MotorControlDevRef"=w215) -> ("error out"=w212:errorcluster, "Output"=w211:dbl)  [unwired: 7 in, 1 out]
            n115 = Greater Or Equal?(x=w206, y=w205) -> (x >= y?=w207:bool)
            n116 = call-poly <vilib>:"NT Write Value.vi"("error in"=w212, "Numeric"=w211, "Name"=" Strafe Motor") -> ()  [unwired: 8 in, 1 out]
            n117 = Wait (ms)(milliseconds to wait=50) -> ()  [unwired: 1 out]
            n118 = call-poly <vilib>:"WPI_RobotDriveArcadeDrive.vi"("Y axis value"=0.0 ("X axis value"), "X axis value"=0.0, "RobotDriveDevRef"=w219) -> ("RobotDriveDevRef"=w222:T11)  [unwired: 1 in, 7 out]
          }
          n119 = while {
            tunnel: [w255] -> w203
            tunnel: w200 -> [w252]
            i -> [w244]
            stop <- w243 stop-if-true
            n120 = call-poly <vilib>:"NT Read Value.vi"("Default Value"=20.0 ("X axis value"), "Name"="Mid Switch Forward Time") -> ("Numeric"=w245:dbl)  [unwired: 8 in, 1 out]
            n121 = Wait (ms)(milliseconds to wait=50) -> ()  [unwired: 1 out]
            n122 = call-poly <vilib>:"NT Read Value.vi"("Default Value"=0.7 ("X axis value"), "Name"="Mid Switch Forward Speed") -> ("Numeric"=w248:dbl)  [unwired: 8 in, 1 out]
            n123 = Negate(x=w248) -> (-x=w247:dbl)
            n124 = Greater Or Equal?(x=w244, y=w245) -> (x >= y?=w243:bool)
            n125 = call-poly <vilib>:"WPI_RobotDriveArcadeDrive.vi"("Y axis value"=w247, "X axis value"=0.0, "RobotDriveDevRef"=w252) -> ("RobotDriveDevRef"=w255:T11)  [unwired: 1 in, 7 out]
          }
          n126 = while {
            tunnel: [w241] -> w202
            tunnel: w203 -> [w237]
            i -> [w223]
            stop <- w240 stop-if-true
            n127 = call <vilib>:"WPI_MotorControlRefNum Registry Get.vi"("refnum name"="Strafe Motor") -> ("MotorControlDevRef"=w235:T12)  [unwired: 9 in, 1 out]
            n128 = call-poly <vilib>:"NT Read Value.vi"("Default Value"=0.9 ("X axis value"), "Name"="Mid Switch Strafe Speed") -> ("Numeric"=w225:dbl)  [unwired: 8 in, 1 out]
            n129 = call-poly <vilib>:"NT Read Value.vi"("Default Value"=90.0 ("X axis value"), "Name"="Mid Switch Strafe Time") -> ("Numeric"=w228:dbl)  [unwired: 8 in, 1 out]
            n130 = call <vilib>:"WPI_MotorControlSetOutput.vi"("Output"=w225, "MotorControlDevRef"=w235) -> ("error out"=w233:errorcluster, "MotorControlDevRef"=w234:T12)  [unwired: 7 in, 1 out]
            n131 = call <vilib>:"WPI_MotorControlGetOutput.vi"("error in"=w233, "MotorControlDevRef"=w234) -> ("error out"=w231:errorcluster, "Output"=w230:dbl)  [unwired: 7 in, 1 out]
            n132 = Greater Or Equal?(x=w223, y=w228) -> (x >= y?=w240:bool)
            n133 = call-poly <vilib>:"WPI_RobotDriveArcadeDrive.vi"("Y axis value"=0.0 ("X axis value"), "X axis value"=0.0, "RobotDriveDevRef"=w237) -> ("RobotDriveDevRef"=w241:T11)  [unwired: 1 in, 7 out]
            n134 = call-poly <vilib>:"NT Write Value.vi"("error in"=w231, "Numeric"=w230, "Name"=" Strafe Motor") -> ()  [unwired: 8 in, 1 out]
            n135 = Wait (ms)(milliseconds to wait=50) -> ()  [unwired: 1 out]
          }
          n136 = while {
            tunnel: w202 -> [w257]
            tunnel: [w256] -> _
            stop <- FALSE stop-if-true
            # "stand still"
            n137 = call-poly <vilib>:"WPI_RobotDriveArcadeDrive.vi"("Y axis value"=0.0 ("X axis value"), "X axis value"=0.0, "RobotDriveDevRef"=w257) -> ("RobotDriveDevRef"=w256:T11)  [unwired: 1 in, 7 out]
            n138 = Wait (ms)(milliseconds to wait=50) -> ()  [unwired: 1 out]
          }
        }
      }
    }
    frame "Switch Mid Reverse" {
      n139 = case shown="\"L\"" w262 {
        frame "R", Default {
          # "5 Seconds"
          n140 = call <vilib>:"WPI_RobotDriveRefNum Registry Get.vi"("refnum name"="Talon SRX") -> ("RobotDriveDevRef"=w266:T11)  [unwired: 1 in, 9 out]
          n141 = while {
            tunnel: [w310] -> w265
            tunnel: w266 -> [w306]
            i -> [w301]
            stop <- w309 stop-if-true
            n142 = call-poly <vilib>:"NT Read Value.vi"("Name"="MSR Slow Time") -> ("Numeric"=w305:dbl)  [unwired: 9 in, 1 out]
            n143 = Wait (ms)(milliseconds to wait=50) -> ()  [unwired: 1 out]
            n144 = call-poly <vilib>:"NT Read Value.vi"("Default Value"=0.7 ("X axis value"), "Name"="MSR Slow Speed") -> ("Numeric"=w300:dbl)  [unwired: 8 in, 1 out]
            n145 = Greater Or Equal?(x=w301, y=w305) -> (x >= y?=w309:bool)
            n146 = call-poly <vilib>:"WPI_RobotDriveArcadeDrive.vi"("Y axis value"=w300, "X axis value"=0.0, "RobotDriveDevRef"=w306) -> ("RobotDriveDevRef"=w310:T11)  [unwired: 1 in, 7 out]
          }
          n147 = while {
            tunnel: [w299] -> w264
            tunnel: w265 -> [w295]
            i -> [w286]
            stop <- w298 stop-if-true
            n148 = call <vilib>:"WPI_MotorControlRefNum Registry Get.vi"("refnum name"="Strafe Motor") -> ("MotorControlDevRef"=w292:T12)  [unwired: 9 in, 1 out]
            n149 = call-poly <vilib>:"NT Read Value.vi"("Default Value"=1.0 ("X axis value"), "Name"="MSR Strafe Speed") -> ("Numeric"=w280:dbl)  [unwired: 8 in, 1 out]
            n150 = call-poly <vilib>:"NT Read Value.vi"("Default Value"=20.0 ("X axis value"), "Name"="MSR Strafe Time") -> ("Numeric"=w283:dbl)  [unwired: 8 in, 1 out]
            n151 = Negate(x=w280) -> (-x=w279:dbl)
            n152 = call <vilib>:"WPI_MotorControlSetOutput.vi"("Output"=w279, "MotorControlDevRef"=w292) -> ("error out"=w290:errorcluster, "MotorControlDevRef"=w291:T12)  [unwired: 7 in, 1 out]
            n153 = call <vilib>:"WPI_MotorControlGetOutput.vi"("error in"=w290, "MotorControlDevRef"=w291) -> ("error out"=w288:errorcluster, "Output"=w287:dbl)  [unwired: 7 in, 1 out]
            n154 = Wait (ms)(milliseconds to wait=50) -> ()  [unwired: 1 out]
            n155 = Greater Or Equal?(x=w286, y=w283) -> (x >= y?=w298:bool)
            n156 = call-poly <vilib>:"NT Write Value.vi"("error in"=w288, "Numeric"=w287, "Name"=" Strafe Motor") -> ()  [unwired: 8 in, 1 out]
            n157 = call-poly <vilib>:"WPI_RobotDriveArcadeDrive.vi"("Y axis value"=0.0 ("X axis value"), "X axis value"=0.0, "RobotDriveDevRef"=w295) -> ("RobotDriveDevRef"=w299:T11)  [unwired: 1 in, 7 out]
          }
          n158 = while {
            tunnel: [w278] -> w263
            tunnel: w264 -> [w274]
            i -> [w269]
            stop <- w277 stop-if-true
            n159 = call-poly <vilib>:"NT Read Value.vi"("Name"="MSR Fast Time") -> ("Numeric"=w273:dbl)  [unwired: 9 in, 1 out]
            n160 = Wait (ms)(milliseconds to wait=50) -> ()  [unwired: 1 out]
            n161 = call-poly <vilib>:"NT Read Value.vi"("Default Value"=0.7 ("X axis value"), "Name"="MSR Fast Speed") -> ("Numeric"=w268:dbl)  [unwired: 8 in, 1 out]
            n162 = Greater Or Equal?(x=w269, y=w273) -> (x >= y?=w277:bool)
            n163 = call-poly <vilib>:"WPI_RobotDriveArcadeDrive.vi"("Y axis value"=w268, "X axis value"=0.0, "RobotDriveDevRef"=w274) -> ("RobotDriveDevRef"=w278:T11)  [unwired: 1 in, 7 out]
          }
          n164 = while {
            tunnel: w263 -> [w312]
            tunnel: [w311] -> _
            stop <- FALSE stop-if-true
            # "stand still"
            n165 = call-poly <vilib>:"WPI_RobotDriveArcadeDrive.vi"("Y axis value"=0.0 ("X axis value"), "X axis value"=0.0, "RobotDriveDevRef"=w312) -> ("RobotDriveDevRef"=w311:T11)  [unwired: 1 in, 7 out]
            n166 = Wait (ms)(milliseconds to wait=50) -> ()  [unwired: 1 out]
          }
        }
        frame "L" {
          # "5 Seconds"
          n167 = call <vilib>:"WPI_RobotDriveRefNum Registry Get.vi"("refnum name"="Talon SRX") -> ("RobotDriveDevRef"=w320:T11)  [unwired: 1 in, 9 out]
          n168 = while {
            tunnel: [w363] -> w319
            tunnel: w320 -> [w359]
            i -> [w354]
            stop <- w362 stop-if-true
            n169 = call-poly <vilib>:"NT Read Value.vi"("Name"="MSR Slow Time") -> ("Numeric"=w358:dbl)  [unwired: 9 in, 1 out]
            n170 = Wait (ms)(milliseconds to wait=50) -> ()  [unwired: 1 out]
            n171 = call-poly <vilib>:"NT Read Value.vi"("Default Value"=0.7 ("X axis value"), "Name"="MSR Slow Speed") -> ("Numeric"=w353:dbl)  [unwired: 8 in, 1 out]
            n172 = Greater Or Equal?(x=w354, y=w358) -> (x >= y?=w362:bool)
            n173 = call-poly <vilib>:"WPI_RobotDriveArcadeDrive.vi"("Y axis value"=w353, "X axis value"=0.0, "RobotDriveDevRef"=w359) -> ("RobotDriveDevRef"=w363:T11)  [unwired: 1 in, 7 out]
          }
          n174 = while {
            tunnel: [w352] -> w318
            tunnel: w319 -> [w348]
            i -> [w339]
            stop <- w351 stop-if-true
            n175 = call <vilib>:"WPI_MotorControlRefNum Registry Get.vi"("refnum name"="Strafe Motor") -> ("MotorControlDevRef"=w345:T12)  [unwired: 9 in, 1 out]
            n176 = call-poly <vilib>:"NT Read Value.vi"("Default Value"=1.0 ("X axis value"), "Name"="MSR Strafe Speed") -> ("Numeric"=w333:dbl)  [unwired: 8 in, 1 out]
            n177 = call-poly <vilib>:"NT Read Value.vi"("Default Value"=20.0 ("X axis value"), "Name"="MSR Strafe Time") -> ("Numeric"=w336:dbl)  [unwired: 8 in, 1 out]
            n178 = call <vilib>:"WPI_MotorControlSetOutput.vi"("Output"=w333, "MotorControlDevRef"=w345) -> ("error out"=w343:errorcluster, "MotorControlDevRef"=w344:T12)  [unwired: 7 in, 1 out]
            n179 = call <vilib>:"WPI_MotorControlGetOutput.vi"("error in"=w343, "MotorControlDevRef"=w344) -> ("error out"=w341:errorcluster, "Output"=w340:dbl)  [unwired: 7 in, 1 out]
            n180 = Wait (ms)(milliseconds to wait=50) -> ()  [unwired: 1 out]
            n181 = Greater Or Equal?(x=w339, y=w336) -> (x >= y?=w351:bool)
            n182 = call-poly <vilib>:"NT Write Value.vi"("error in"=w341, "Numeric"=w340, "Name"=" Strafe Motor") -> ()  [unwired: 8 in, 1 out]
            n183 = call-poly <vilib>:"WPI_RobotDriveArcadeDrive.vi"("Y axis value"=0.0 ("X axis value"), "X axis value"=0.0, "RobotDriveDevRef"=w348) -> ("RobotDriveDevRef"=w352:T11)  [unwired: 1 in, 7 out]
          }
          n184 = while {
            tunnel: [w332] -> w317
            tunnel: w318 -> [w328]
            i -> [w323]
            stop <- w331 stop-if-true
            n185 = call-poly <vilib>:"NT Read Value.vi"("Name"="MSR Fast Time") -> ("Numeric"=w327:dbl)  [unwired: 9 in, 1 out]
            n186 = Wait (ms)(milliseconds to wait=50) -> ()  [unwired: 1 out]
            n187 = call-poly <vilib>:"NT Read Value.vi"("Default Value"=0.7 ("X axis value"), "Name"="MSR Fast Speed") -> ("Numeric"=w322:dbl)  [unwired: 8 in, 1 out]
            n188 = Greater Or Equal?(x=w323, y=w327) -> (x >= y?=w331:bool)
            n189 = call-poly <vilib>:"WPI_RobotDriveArcadeDrive.vi"("Y axis value"=w322, "X axis value"=0.0, "RobotDriveDevRef"=w328) -> ("RobotDriveDevRef"=w332:T11)  [unwired: 1 in, 7 out]
          }
          n190 = while {
            tunnel: w317 -> [w365]
            tunnel: [w364] -> _
            stop <- FALSE stop-if-true
            # "stand still"
            n191 = call-poly <vilib>:"WPI_RobotDriveArcadeDrive.vi"("Y axis value"=0.0 ("X axis value"), "X axis value"=0.0, "RobotDriveDevRef"=w365) -> ("RobotDriveDevRef"=w364:T11)  [unwired: 1 in, 7 out]
            n192 = Wait (ms)(milliseconds to wait=50) -> ()  [unwired: 1 out]
          }
        }
      }
    }
    frame "Switch Mid Reverse Direct" {
      n193 = case shown="\"R\", Default" w370 {
        frame "L" {
          # "5 Seconds"
          n194 = call <vilib>:"WPI_RobotDriveRefNum Registry Get.vi"("refnum name"="Talon SRX") -> ("RobotDriveDevRef"=w373:T11)  [unwired: 1 in, 9 out]
          n195 = while {
            tunnel: [w406] -> w371
            tunnel: w373 -> [w402]
            i -> [w397]
            stop <- w405 stop-if-true
            n196 = call <vilib>:"WPI_MotorControlRefNum Registry Get.vi"("refnum name"="Strafe Motor") -> ("MotorControlDevRef"=w392:T12)  [unwired: 9 in, 1 out]
            n197 = call-poly <vilib>:"NT Read Value.vi"("Name"="MSR Slow Time") -> ("Numeric"=w401:dbl)  [unwired: 9 in, 1 out]
            n198 = Wait (ms)(milliseconds to wait=50) -> ()  [unwired: 1 out]
            n199 = call-poly <vilib>:"NT Read Value.vi"("Default Value"=0.7 ("X axis value"), "Name"="MSR Slow Speed") -> ("Numeric"=w396:dbl)  [unwired: 8 in, 1 out]
            n200 = call-poly <vilib>:"NT Read Value.vi"("Default Value"=1.0 ("X axis value"), "Name"="MSR Strafe Speed") -> ("Numeric"=w386:dbl)  [unwired: 8 in, 1 out]
            n201 = call <vilib>:"WPI_MotorControlSetOutput.vi"("Output"=w386, "MotorControlDevRef"=w392) -> ("error out"=w390:errorcluster, "MotorControlDevRef"=w391:T12)  [unwired: 7 in, 1 out]
            n202 = call <vilib>:"WPI_MotorControlGetOutput.vi"("error in"=w390, "MotorControlDevRef"=w391) -> ("error out"=w388:errorcluster, "Output"=w387:dbl)  [unwired: 7 in, 1 out]
            n203 = Greater Or Equal?(x=w397, y=w401) -> (x >= y?=w405:bool)
            n204 = call-poly <vilib>:"NT Write Value.vi"("error in"=w388, "Numeric"=w387, "Name"=" Strafe Motor") -> ()  [unwired: 8 in, 1 out]
            n205 = call-poly <vilib>:"WPI_RobotDriveArcadeDrive.vi"("Y axis value"=w396, "X axis value"=0.0, "RobotDriveDevRef"=w402) -> ("RobotDriveDevRef"=w406:T11)  [unwired: 1 in, 7 out]
          }
          n206 = while {
            tunnel: [w385] -> w372
            tunnel: w371 -> [w381]
            i -> [w376]
            stop <- w384 stop-if-true
            n207 = call-poly <vilib>:"NT Read Value.vi"("Name"="MSR Fast Time") -> ("Numeric"=w380:dbl)  [unwired: 9 in, 1 out]
            n208 = Wait (ms)(milliseconds to wait=50) -> ()  [unwired: 1 out]
            n209 = call-poly <vilib>:"NT Read Value.vi"("Default Value"=0.7 ("X axis value"), "Name"="MSR Fast Speed") -> ("Numeric"=w375:dbl)  [unwired: 8 in, 1 out]
            n210 = Greater Or Equal?(x=w376, y=w380) -> (x >= y?=w384:bool)
            n211 = call-poly <vilib>:"WPI_RobotDriveArcadeDrive.vi"("Y axis value"=w375, "X axis value"=0.0, "RobotDriveDevRef"=w381) -> ("RobotDriveDevRef"=w385:T11)  [unwired: 1 in, 7 out]
          }
          n212 = while {
            tunnel: w372 -> [w408]
            tunnel: [w407] -> _
            stop <- FALSE stop-if-true
            # "stand still"
            n213 = call-poly <vilib>:"WPI_RobotDriveArcadeDrive.vi"("Y axis value"=0.0 ("X axis value"), "X axis value"=0.0, "RobotDriveDevRef"=w408) -> ("RobotDriveDevRef"=w407:T11)  [unwired: 1 in, 7 out]
            n214 = Wait (ms)(milliseconds to wait=50) -> ()  [unwired: 1 out]
          }
        }
        frame "R", Default {
          # "5 Seconds"
          n215 = call <vilib>:"WPI_RobotDriveRefNum Registry Get.vi"("refnum name"="Talon SRX") -> ("RobotDriveDevRef"=w415:T11)  [unwired: 1 in, 9 out]
          n216 = while {
            tunnel: [w449] -> w413
            tunnel: w415 -> [w445]
            i -> [w440]
            stop <- w448 stop-if-true
            n217 = call <vilib>:"WPI_MotorControlRefNum Registry Get.vi"("refnum name"="Strafe Motor") -> ("MotorControlDevRef"=w435:T12)  [unwired: 9 in, 1 out]
            n218 = call-poly <vilib>:"NT Read Value.vi"("Name"="MSR Slow Time") -> ("Numeric"=w444:dbl)  [unwired: 9 in, 1 out]
            n219 = Wait (ms)(milliseconds to wait=50) -> ()  [unwired: 1 out]
            n220 = call-poly <vilib>:"NT Read Value.vi"("Default Value"=0.7 ("X axis value"), "Name"="MSR Slow Speed") -> ("Numeric"=w439:dbl)  [unwired: 8 in, 1 out]
            n221 = call-poly <vilib>:"NT Read Value.vi"("Default Value"=1.0 ("X axis value"), "Name"="MSR Strafe Speed") -> ("Numeric"=w429:dbl)  [unwired: 8 in, 1 out]
            n222 = Greater Or Equal?(x=w440, y=w444) -> (x >= y?=w448:bool)
            n223 = Negate(x=w429) -> (-x=w428:dbl)
            n224 = call <vilib>:"WPI_MotorControlSetOutput.vi"("Output"=w428, "MotorControlDevRef"=w435) -> ("error out"=w433:errorcluster, "MotorControlDevRef"=w434:T12)  [unwired: 7 in, 1 out]
            n225 = call <vilib>:"WPI_MotorControlGetOutput.vi"("error in"=w433, "MotorControlDevRef"=w434) -> ("error out"=w431:errorcluster, "Output"=w430:dbl)  [unwired: 7 in, 1 out]
            n226 = call-poly <vilib>:"NT Write Value.vi"("error in"=w431, "Numeric"=w430, "Name"=" Strafe Motor") -> ()  [unwired: 8 in, 1 out]
            n227 = call-poly <vilib>:"WPI_RobotDriveArcadeDrive.vi"("Y axis value"=w439, "X axis value"=0.0, "RobotDriveDevRef"=w445) -> ("RobotDriveDevRef"=w449:T11)  [unwired: 1 in, 7 out]
          }
          n228 = while {
            tunnel: [w427] -> w414
            tunnel: w413 -> [w423]
            i -> [w418]
            stop <- w426 stop-if-true
            n229 = call-poly <vilib>:"NT Read Value.vi"("Name"="MSR Fast Time") -> ("Numeric"=w422:dbl)  [unwired: 9 in, 1 out]
            n230 = Wait (ms)(milliseconds to wait=50) -> ()  [unwired: 1 out]
            n231 = call-poly <vilib>:"NT Read Value.vi"("Default Value"=0.7 ("X axis value"), "Name"="MSR Fast Speed") -> ("Numeric"=w417:dbl)  [unwired: 8 in, 1 out]
            n232 = Greater Or Equal?(x=w418, y=w422) -> (x >= y?=w426:bool)
            n233 = call-poly <vilib>:"WPI_RobotDriveArcadeDrive.vi"("Y axis value"=w417, "X axis value"=0.0, "RobotDriveDevRef"=w423) -> ("RobotDriveDevRef"=w427:T11)  [unwired: 1 in, 7 out]
          }
          n234 = while {
            tunnel: w414 -> [w451]
            tunnel: [w450] -> _
            stop <- FALSE stop-if-true
            # "stand still"
            n235 = call-poly <vilib>:"WPI_RobotDriveArcadeDrive.vi"("Y axis value"=0.0 ("X axis value"), "X axis value"=0.0, "RobotDriveDevRef"=w451) -> ("RobotDriveDevRef"=w450:T11)  [unwired: 1 in, 7 out]
            n236 = Wait (ms)(milliseconds to wait=50) -> ()  [unwired: 1 out]
          }
        }
      }
    }
    frame "Scale Mid" {
      n237 = call <vilib>:"WPI_RobotDriveRefNum Registry Get.vi"("refnum name"="Talon SRX") -> ("RobotDriveDevRef"=w457:T11)  [unwired: 1 in, 9 out]
      n238 = case shown="\"R\", Default" w456 {
        tunnel: w457 -> [w555 _]
        frame "R", Default {
          n239 = call-poly <vilib>:"NT Read Value.vi"("Default Value"=0.5 ("X axis value"), "Name"="FS1_SCA_M_R") -> ("Numeric"=w549:dbl)  [unwired: 8 in, 1 out]
          n240 = call-poly <vilib>:"NT Read Value.vi"("Default Value"=10.0 ("X axis value"), "Name"="FT1_SCA_M_R") -> ("Numeric"=w550:dbl)  [unwired: 8 in, 1 out]
          n241 = call "Auto_timed_forward.vi"("Speed"=w549, "Time"=w550, "RobotDriveDevRef in"=w555) -> ("RobotDriveDevRef"=w554:T11)  [unwired: 2 in]
          n242 = call-poly <vilib>:"NT Read Value.vi"("Default Value"=0.2 ("X axis value"), "Name"="FS3_SCA_M_R") -> ("Numeric"=w529:dbl)  [unwired: 8 in, 1 out]
          n243 = call-poly <vilib>:"NT Read Value.vi"("Default Value"=3.0 ("X axis value"), "Name"="FT3_SCA_M_R") -> ("Numeric"=w526:dbl)  [unwired: 8 in, 1 out]
          n244 = call-poly <vilib>:"NT Read Value.vi"("Default Value"=1.0 ("X axis value"), "Name"="CIS1_SCA_M_R") -> ("Numeric"=w505:dbl)  [unwired: 8 in, 1 out]
          n245 = call-poly <vilib>:"NT Read Value.vi"("Default Value"=40.0 ("X axis value"), "Name"="ST1_SCA_M_R") -> ("Numeric"=w563:dbl)  [unwired: 8 in, 1 out]
          n246 = call-poly <vilib>:"NT Read Value.vi"("Default Value"=10.0 ("X axis value"), "Name"="CIT1_SCA_M_R") -> ("Numeric"=w506:dbl)  [unwired: 8 in, 1 out]
          n247 = call-poly <vilib>:"NT Read Value.vi"("Default Value"=0.7 ("X axis value"), "Name"="SS1_SCA_M_R") -> ("Numeric"=w562:dbl)  [unwired: 8 in, 1 out]
          n248 = call "Auto_timed_strafe.vi"("Strafe Speed"=w562, "Strafe Time"=w563, "RobotDriveDevRef in"=w554) -> ("RobotDriveDevRef out"=w561:T11)  [unwired: 2 in]
          n249 = call-poly <vilib>:"NT Read Value.vi"("Default Value"=-0.2 ("X axis value"), "Name"="FS4_SCA_M_R") -> ("Numeric"=w522:dbl)  [unwired: 8 in, 1 out]
          n250 = call-poly <vilib>:"NT Read Value.vi"("Default Value"=3.0 ("X axis value"), "Name"="FT4_SCA_M_R") -> ("Numeric"=w520:dbl)  [unwired: 8 in, 1 out]
          n251 = call-poly <vilib>:"NT Read Value.vi"("Default Value"=20.0 ("X axis value"), "Name"="FT2_SCA_M_R") -> ("Numeric"=w556:dbl)  [unwired: 8 in, 1 out]
          n252 = call-poly <vilib>:"NT Read Value.vi"("Default Value"=0.7 ("X axis value"), "Name"="FS2_SCA_M_R") -> ("Numeric"=w558:dbl)  [unwired: 8 in, 1 out]
          n253 = call "Auto_timed_forward.vi"("Speed"=w558, "Time"=w556, "RobotDriveDevRef in"=w561) -> ("RobotDriveDevRef"=w542:T11)  [unwired: 2 in]
          n254 = call-poly <vilib>:"NT Read Value.vi"("Default Value"=5.0 ("X axis value"), "Name"="CLT2_SCA_M_R") -> ("Numeric"=w514:dbl)  [unwired: 8 in, 1 out]
          n255 = call-poly <vilib>:"NT Read Value.vi"("Default Value"=-0.4 ("X axis value"), "Name"="CLS2_SCA_M_R") -> ("Numeric"=w515:dbl)  [unwired: 8 in, 1 out]
          n256 = call-poly <vilib>:"NT Read Value.vi"("Default Value"=10.0 ("X axis value"), "Name"="ST2_SCA_M_R") -> ("Numeric"=w544:dbl)  [unwired: 8 in, 1 out]
          n257 = call-poly <vilib>:"NT Read Value.vi"("Default Value"=-0.5 ("X axis value"), "Name"="SS2_SCA_M_R") -> ("Numeric"=w543:dbl)  [unwired: 8 in, 1 out]
          n258 = call "Auto_timed_strafe.vi"("Strafe Speed"=w543, "Strafe Time"=w544, "RobotDriveDevRef in"=w542) -> ("RobotDriveDevRef out"=w541:T11)  [unwired: 2 in]
          n259 = call-poly <vilib>:"NT Read Value.vi"("Default Value"=10.0 ("X axis value"), "Name"="TTT1_SCA_M_R") -> ("Numeric"=w499:dbl)  [unwired: 8 in, 1 out]
          n260 = call-poly <vilib>:"NT Read Value.vi"("Default Value"=-0.5 ("X axis value"), "Name"="TTS1_SCA_M_R") -> ("Numeric"=w500:dbl)  [unwired: 8 in, 1 out]
          n261 = call-poly <vilib>:"NT Read Value.vi"("Default Value"=5.0 ("X axis value"), "Name"="CLT1_SCA_M_R") -> ("Numeric"=w536:dbl)  [unwired: 8 in, 1 out]
          n262 = call-poly <vilib>:"NT Read Value.vi"("Default Value"=0.6 ("X axis value"), "Name"="CLS1_SCA_M_R") -> ("Numeric"=w535:dbl)  [unwired: 8 in, 1 out]
          n263 = call-poly <vilib>:"NT Read Value.vi"("Default Value"=0.25 ("X axis value"), "Name"="CIDS1_SCA_M_R") -> ("Numeric"=w488:dbl)  [unwired: 8 in, 1 out]
          n264 = call "Auto_timed_cube lift.vi"("Cube Lift Speed"=w535, "Cube Lift Time"=w536, "RobotDriveDevRef in"=w541) -> ("RobotDriveDevRef out"=w527:T11)  [unwired: 2 in]
          n265 = call "Auto_timed_forward.vi"("Speed"=w529, "Time"=w526, "RobotDriveDevRef in"=w527) -> ("RobotDriveDevRef"=w512:T11)  [unwired: 2 in]
          n266 = call "Auto_timed_cube in.vi"("Cube In Speed"=w505, "Cube In Time"=w506, "RobotDriveDevRef in"=w512) -> ("RobotDriveDevRef out"=w511:T11)  [unwired: 2 in]
          n267 = call "Auto_timed_forward.vi"("Speed"=w522, "Time"=w520, "RobotDriveDevRef in"=w511) -> ("RobotDriveDevRef"=w513:T11)  [unwired: 2 in]
          n268 = call "Auto_timed_cube lift.vi"("Cube Lift Speed"=w515, "Cube Lift Time"=w514, "RobotDriveDevRef in"=w513) -> ("RobotDriveDevRef out"=w498:T11)  [unwired: 2 in]
          n269 = call "Auto_timed_turn.vi"("Speed"=w500, "Time"=w499, "RobotDriveDevRef in"=w498) -> ("RobotDriveDevRef"=w492:T11)  [unwired: 2 in]
          n270 = call-poly <vilib>:"NT Read Value.vi"("Default Value"=1.0 ("X axis value"), "Name"="CIS2_SCA_M_R") -> ("Numeric"=w494:dbl)  [unwired: 8 in, 1 out]
          n271 = call-poly <vilib>:"NT Read Value.vi"("Default Value"=10.0 ("X axis value"), "Name"="CIT2_SCA_M_R") -> ("Numeric"=w493:dbl)  [unwired: 8 in, 1 out]
          n272 = call "Auto_timed_cube in+drive.vi"("Cube In Speed"=w494, "Cube In Time"=w493, "Drive Speed"=w488, "RobotDriveDevRef in"=w492) -> ("RobotDriveDevRef out"=w481:T11)  [unwired: 1 in]
          n273 = call-poly <vilib>:"NT Read Value.vi"("Default Value"=-0.25 ("X axis value"), "Name"="FS5_SCA_M_R") -> ("Numeric"=w484:dbl)  [unwired: 8 in, 1 out]
          n274 = call-poly <vilib>:"NT Read Value.vi"("Default Value"=10.0 ("X axis value"), "Name"="FT5_SCA_M_R") -> ("Numeric"=w482:dbl)  [unwired: 8 in, 1 out]
          n275 = call "Auto_timed_forward.vi"("Speed"=w484, "Time"=w482, "RobotDriveDevRef in"=w481) -> ("RobotDriveDevRef"=w474:T11)  [unwired: 2 in]
          n276 = call-poly <vilib>:"NT Read Value.vi"("Default Value"=10.0 ("X axis value"), "Name"="TTT2_SCA_M_R") -> ("Numeric"=w475:dbl)  [unwired: 8 in, 1 out]
          n277 = call-poly <vilib>:"NT Read Value.vi"("Default Value"=0.5 ("X axis value"), "Name"="TTS2_SCA_M_R") -> ("Numeric"=w476:dbl)  [unwired: 8 in, 1 out]
          n278 = call "Auto_timed_turn.vi"("Speed"=w476, "Time"=w475, "RobotDriveDevRef in"=w474) -> ("RobotDriveDevRef"=w467:T11)  [unwired: 2 in]
          n279 = call-poly <vilib>:"NT Read Value.vi"("Default Value"=5.0 ("X axis value"), "Name"="CLT3_SCA_M_R") -> ("Numeric"=w468:dbl)  [unwired: 8 in, 1 out]
          n280 = call-poly <vilib>:"NT Read Value.vi"("Default Value"=0.6 ("X axis value"), "Name"="CLS3_SCA_M_R") -> ("Numeric"=w469:dbl)  [unwired: 8 in, 1 out]
          n281 = call "Auto_timed_cube lift.vi"("Cube Lift Speed"=w469, "Cube Lift Time"=w468, "RobotDriveDevRef in"=w467) -> ("RobotDriveDevRef out"=w460:T11)  [unwired: 2 in]
          n282 = call-poly <vilib>:"NT Read Value.vi"("Default Value"=1.0 ("X axis value"), "Name"="CIS2_SCA_M_R") -> ("Numeric"=w461:dbl)  [unwired: 8 in, 1 out]
          n283 = call-poly <vilib>:"NT Read Value.vi"("Default Value"=10.0 ("X axis value"), "Name"="CIT2_SCA_M_R") -> ("Numeric"=w462:dbl)  [unwired: 8 in, 1 out]
          n284 = call "Auto_timed_cube in.vi"("Cube In Speed"=w461, "Cube In Time"=w462, "RobotDriveDevRef in"=w460) -> ("RobotDriveDevRef out"=w459:T11)  [unwired: 2 in]
          n285 = while {
            tunnel: w459 -> [w569]
            tunnel: [w568] -> _
            stop <- FALSE stop-if-true
            # "stand still"
            n286 = call-poly <vilib>:"WPI_RobotDriveArcadeDrive.vi"("Y axis value"=0.0 ("X axis value"), "X axis value"=0.0, "RobotDriveDevRef"=w569) -> ("RobotDriveDevRef"=w568:T11)  [unwired: 1 in, 7 out]
            n287 = Wait (ms)(milliseconds to wait=50) -> ()  [unwired: 1 out]
          }
        }
        frame "L" {
          # "5 Seconds"
          n288 = call <vilib>:"WPI_RobotDriveRefNum Registry Get.vi"("refnum name"="Talon SRX") -> ("RobotDriveDevRef"=w578:T11)  [unwired: 1 in, 9 out]
          n289 = call-poly <vilib>:"NT Read Value.vi"("Default Value"=0.5 ("X axis value"), "Name"="Strafe From Wall Speed") -> ("Numeric"=w574:dbl)  [unwired: 8 in, 1 out]
          n290 = while {
            tunnel: [w599] -> w577
            tunnel: w578 -> [w596]
            tunnel: w574 -> [w587]
            i -> [w583]
            stop <- w584 stop-if-true
            n291 = call <vilib>:"WPI_MotorControlRefNum Registry Get.vi"("refnum name"="Strafe Motor") -> ("MotorControlDevRef"=w593:T12)  [unwired: 9 in, 1 out]
            n292 = call-poly <vilib>:"NT Read Value.vi"("Default Value"=20.0 ("X axis value"), "Name"="Strafe From Wall Time") -> ("Numeric"=w582:dbl)  [unwired: 8 in, 1 out]
            n293 = call <vilib>:"WPI_MotorControlSetOutput.vi"("Output"=w587, "MotorControlDevRef"=w593) -> ("error out"=w591:errorcluster, "MotorControlDevRef"=w592:T12)  [unwired: 7 in, 1 out]
            n294 = call <vilib>:"WPI_MotorControlGetOutput.vi"("error in"=w591, "MotorControlDevRef"=w592) -> ("error out"=w589:errorcluster, "Output"=w588:dbl)  [unwired: 7 in, 1 out]
            n295 = Greater Or Equal?(x=w583, y=w582) -> (x >= y?=w584:bool)
            n296 = call-poly <vilib>:"NT Write Value.vi"("error in"=w589, "Numeric"=w588, "Name"=" Strafe Motor") -> ()  [unwired: 8 in, 1 out]
            n297 = Wait (ms)(milliseconds to wait=50) -> ()  [unwired: 1 out]
            n298 = call-poly <vilib>:"WPI_RobotDriveArcadeDrive.vi"("Y axis value"=0.0 ("X axis value"), "X axis value"=0.0, "RobotDriveDevRef"=w596) -> ("RobotDriveDevRef"=w599:T11)  [unwired: 1 in, 7 out]
          }
          n299 = while {
            tunnel: [w632] -> w580
            tunnel: w577 -> [w629]
            i -> [w621]
            stop <- w620 stop-if-true
            n300 = call-poly <vilib>:"NT Read Value.vi"("Default Value"=20.0 ("X axis value"), "Name"="Mid Switch Forward Time") -> ("Numeric"=w622:dbl)  [unwired: 8 in, 1 out]
            n301 = Wait (ms)(milliseconds to wait=50) -> ()  [unwired: 1 out]
            n302 = call-poly <vilib>:"NT Read Value.vi"("Default Value"=0.7 ("X axis value"), "Name"="Mid Switch Forward Speed") -> ("Numeric"=w625:dbl)  [unwired: 8 in, 1 out]
            n303 = Negate(x=w625) -> (-x=w624:dbl)
            n304 = Greater Or Equal?(x=w621, y=w622) -> (x >= y?=w620:bool)
            n305 = call-poly <vilib>:"WPI_RobotDriveArcadeDrive.vi"("Y axis value"=w624, "X axis value"=0.0, "RobotDriveDevRef"=w629) -> ("RobotDriveDevRef"=w632:T11)  [unwired: 1 in, 7 out]
          }
          n306 = while {
            tunnel: [w618] -> w579
            tunnel: w580 -> [w614]
            i -> [w600]
            stop <- w617 stop-if-true
            n307 = call <vilib>:"WPI_MotorControlRefNum Registry Get.vi"("refnum name"="Strafe Motor") -> ("MotorControlDevRef"=w612:T12)  [unwired: 9 in, 1 out]
            n308 = call-poly <vilib>:"NT Read Value.vi"("Default Value"=0.9 ("X axis value"), "Name"="Mid Switch Strafe Speed") -> ("Numeric"=w602:dbl)  [unwired: 8 in, 1 out]
            n309 = call-poly <vilib>:"NT Read Value.vi"("Default Value"=90.0 ("X axis value"), "Name"="Mid Switch Strafe Time") -> ("Numeric"=w605:dbl)  [unwired: 8 in, 1 out]
            n310 = call <vilib>:"WPI_MotorControlSetOutput.vi"("Output"=w602, "MotorControlDevRef"=w612) -> ("error out"=w610:errorcluster, "MotorControlDevRef"=w611:T12)  [unwired: 7 in, 1 out]
            n311 = call <vilib>:"WPI_MotorControlGetOutput.vi"("error in"=w610, "MotorControlDevRef"=w611) -> ("error out"=w608:errorcluster, "Output"=w607:dbl)  [unwired: 7 in, 1 out]
            n312 = Greater Or Equal?(x=w600, y=w605) -> (x >= y?=w617:bool)
            n313 = call-poly <vilib>:"WPI_RobotDriveArcadeDrive.vi"("Y axis value"=0.0 ("X axis value"), "X axis value"=0.0, "RobotDriveDevRef"=w614) -> ("RobotDriveDevRef"=w618:T11)  [unwired: 1 in, 7 out]
            n314 = call-poly <vilib>:"NT Write Value.vi"("error in"=w608, "Numeric"=w607, "Name"=" Strafe Motor") -> ()  [unwired: 8 in, 1 out]
            n315 = Wait (ms)(milliseconds to wait=50) -> ()  [unwired: 1 out]
          }
          n316 = while {
            tunnel: w579 -> [w634]
            tunnel: [w633] -> _
            stop <- FALSE stop-if-true
            # "stand still"
            n317 = call-poly <vilib>:"WPI_RobotDriveArcadeDrive.vi"("Y axis value"=0.0 ("X axis value"), "X axis value"=0.0, "RobotDriveDevRef"=w634) -> ("RobotDriveDevRef"=w633:T11)  [unwired: 1 in, 7 out]
            n318 = Wait (ms)(milliseconds to wait=50) -> ()  [unwired: 1 out]
          }
        }
      }
    }
    frame "Ultrasonic PID Test" {
      n319 = disable-structure shown="Disabled" {
        frame Disabled {
          n320 = while {
            stop <- FALSE stop-if-true
            # "P\nI\nD"
            n321 = call-poly <vilib>:"WPI_UltrasonicRefNum Registry Get.vi"("refnum name"="Ultrasonic") -> ("SonarMB1010AnalogDevRef"=w663:T17)  [unwired: 9 in, 1 out]
            n322 = call-poly <vilib>:"WPI_UltrasonicGetRange.vi"("SonarMB1010AnalogDevRef"=w663) -> ("Distance"=w662:dbl)  [unwired: 8 in, 2 out]
            n323 = Wait (ms)(milliseconds to wait=u32 20) -> ()  [unwired: 1 out]
            n324 = Add(x=w662, y=0.58558) -> (x+y=w660:dbl)
            n325 = Divide(x=w660, y=1.2003) -> (x/y=w641:dbl)
            n326 = call-poly <vilib>:"NT Read Value.vi"("Default Value"=15.0, "Name"="Target Distance" ("refnum name")) -> ("Numeric"=w640:dbl)  [unwired: 8 in, 1 out]
            n327 = Bundle("P"=0.3, "I"=10.0, "D"=0.0) -> (w644:cluster{"P":dbl, "I":dbl, "D":dbl})  [unwired: 1 in]
            n328 = call-poly <vilib>:"PID.vi"("output range"=cluster{"Lower value":sgl, "Upper value":sgl} {"Lower value"=-1.0, "Upper value"=1.0} ("Range"), "dt (s)"=0.01, "PID gains"=w644, "process variable"=w641, "setpoint"=w640) -> ("output"=w639:dbl)  [unwired: 5 in, 1 out]
            n329 = disable-structure shown="Disabled" {
              disable-tunnel: w639 -> [w665 _]
              frame Disabled {
                n330 = call <vilib>:"WPI_RobotDriveRefNum Registry Get.vi"("refnum name"="Left and Right Motors") -> ("RobotDriveDevRef"=w667:T11)  [unwired: 1 in, 9 out]
                n331 = call-poly <vilib>:"WPI_RobotDriveArcadeDrive.vi"("Y axis value"=w665, "X axis value"=0.0, "RobotDriveDevRef"=w667) -> ()  [unwired: 1 in, 8 out]
              }
              frame Enabled {
              }
            }
            n332 = call-poly <vilib>:"NT Write Value.vi"("Numeric"=w641, "Name"="Ultrasonic Distance" ("refnum name")) -> ()  [unwired: 9 in, 1 out]
            n333 = call <vilib>:"WPI_MotorControlRefNum Registry Get.vi"("refnum name"="Cube Intake Left") -> ("MotorControlDevRef"=w653:T12)  [unwired: 9 in, 1 out]
            n334 = call <vilib>:"WPI_MotorControlRefNum Registry Get.vi"("refnum name"="Cube Intake Right") -> ("MotorControlDevRef"=w656:T12)  [unwired: 9 in, 1 out]
            n335 = call <vilib>:"WPI_MotorControlSetOutput.vi"("Output"=w639, "MotorControlDevRef"=w653) -> ("MotorControlDevRef"=w654:T12)  [unwired: 7 in, 2 out]
            n336 = call <vilib>:"WPI_MotorControlSetOutput.vi"("Output"=w639, "MotorControlDevRef"=w656) -> ("MotorControlDevRef"=w655:T12)  [unwired: 7 in, 2 out]
            n337 = call <vilib>:"WPI_MotorControlGetOutput.vi"("MotorControlDevRef"=w654) -> ()  [unwired: 8 in, 3 out]
            n338 = call <vilib>:"WPI_MotorControlGetOutput.vi"("MotorControlDevRef"=w655) -> ()  [unwired: 8 in, 3 out]
          }
        }
        frame Enabled {
        }
      }
    }
  }
  n339 = call-poly <vilib>:"NT Read Value.vi"("Name"="Auto Starting Position Options") -> ("String"=w14:string)  [unwired: 9 in, 1 out]
  n340 = call-poly <vilib>:"NT Read Value.vi"("Name"="Auto Starting Position Options") -> ("String"=w11:string)  [unwired: 9 in, 1 out]
  n341 = call-poly <vilib>:"NT Write Value.vi"("String"=w14, "Name"="Alliance Teammate 1 Starting Position") -> ()  [unwired: 9 in, 1 out]
  n342 = call-poly <vilib>:"NT Write Value.vi"("String"=w11, "Name"="Alliance Teammate 2 Starting Position") -> ()  [unwired: 9 in, 1 out]
  n343 = call-poly <vilib>:"NT Read Value.vi"("Name"="Auto Teammate Move Options") -> ("String"=w8:string)  [unwired: 9 in, 1 out]
  n344 = call-poly <vilib>:"NT Read Value.vi"("Name"="Auto Teammate Move Options") -> ("String"=w5:string)  [unwired: 9 in, 1 out]
  n345 = call-poly <vilib>:"NT Write Value.vi"("String"=w8, "Name"="Alliance Teammate 1 Auto Move") -> ()  [unwired: 9 in, 1 out]
  n346 = call-poly <vilib>:"NT Write Value.vi"("String"=w5, "Name"="Alliance Teammate 2 Auto Move") -> ()  [unwired: 9 in, 1 out]
